vi "QImaging_Main.vi"() -> ()   [LabVIEW 2014]
uses:
  QImaging_Basic/Controls/Parameter.ctl
  Release/QImaging.dll
  QImaging_Basic/Controls/Readout Speed.ctl
panel:
  out "dy":dbl
  in  "Readout Speed":T1
  out "Message":string
  in  "Stop Live Preview":bool
  in  "Abort Multi Grab":bool
  in  "Multi Grab":bool
  out "Saturating?":bool
  out "Average":dbl
  out "Std Dev":dbl
  in  "Overwrite?":bool
  in  "Snap current Data":bool
  in  "Save Data":bool
  in  "Racine chemin de sauvegarde":path=path "C:/Users/loa/Documents/DONNEES MANIP GAZ/Hiver 2015"
  out "Warning":bool
  out "Message":string
  in  "Indice":u32
  in  "Nom":string="tir"
  in  "Mode de Sauvegarde":u16(ring)=1 items=["Manuel", "Automatique"]
  out "Max Val":u16
  out "Captured Image":u16[][](graph)
  out "CCD Height":u32=1 min=1 max=4 step=1
  out "CCD Width":u32=1 min=1 max=4 step=1
  out "Camera Handle":u32
  in  "Abort Frame":bool
  out "sizeOfBuf":u32
  out "errcode":i32
  out "pBuf address":u32
  out "pFrame address":u32
  out "Waiting for Trigger":bool
  in  "Grab Image":bool
  in  "Queue Frame":bool
  in  "Trig":bool
  out "ROI Height":u32=1 min=1 max=4 step=1
  out "ROI Width":u32=1 min=1 max=4 step=1
  in  "Binning":u32=1 min=1 max=4 step=1
  out "ParamVal":u32[](array[numeric])
  out "Open Cam Error":i32
  out "LibCam Error":u32
  out "LibOpen error":i32
  in  "Exposure Time (µs)":u32=100
  out "Camera Id":u32
  out "error out":errorcluster
  in  "error in (no error)":errorcluster
  in  "Stop":bool
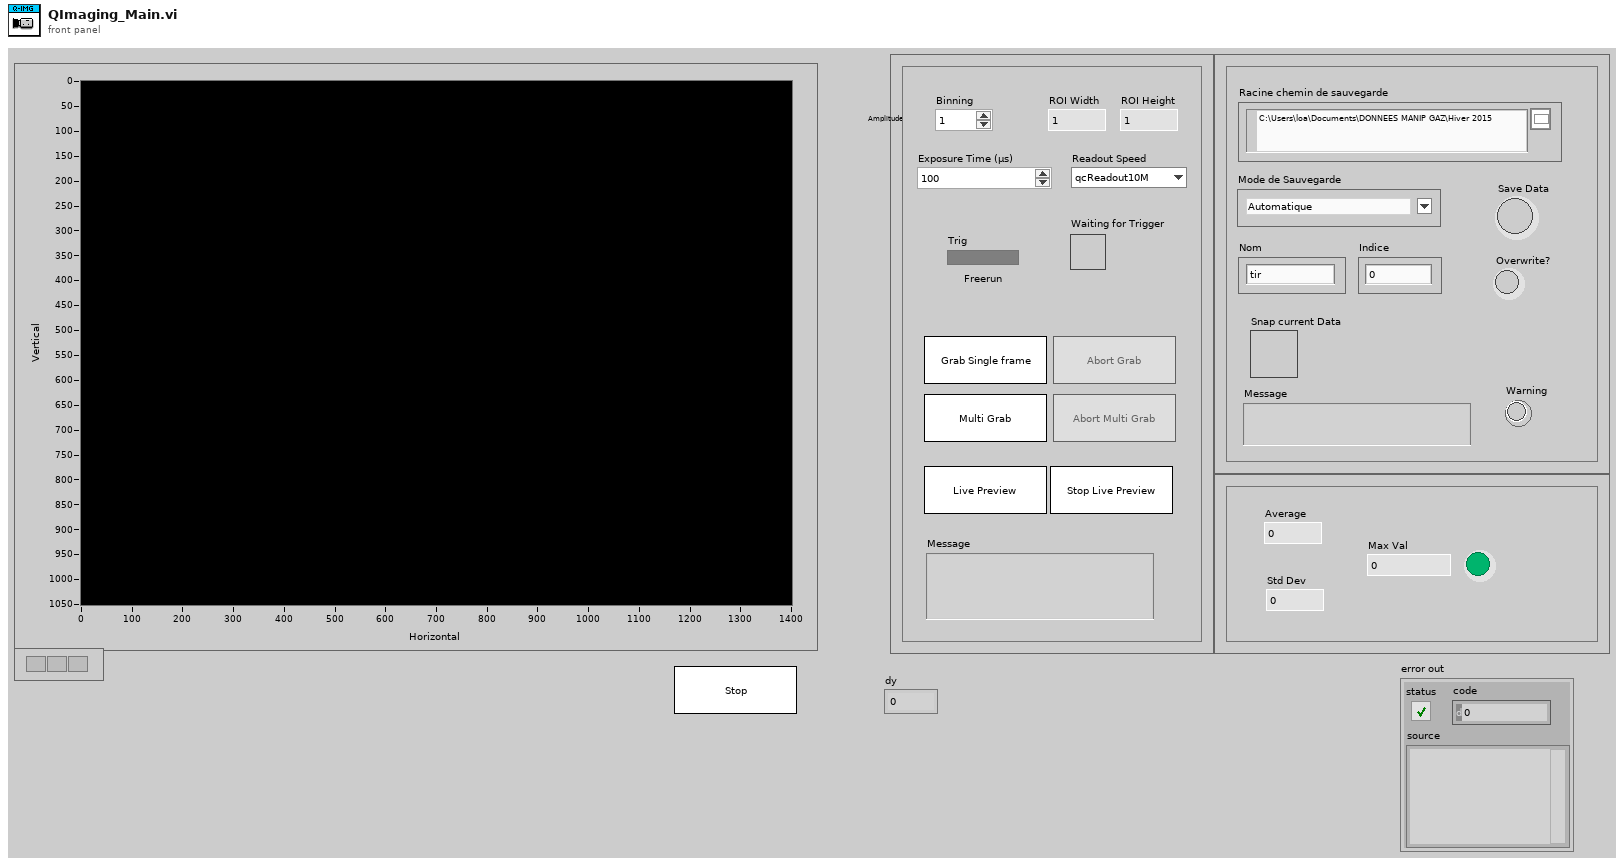
[diagram p1: front panel]
types:
  T1 = typedef "Readout Speed.ctl" = enum16{"qcReadout10M", "qcReadout20M", "qcReadout30M"}
  T2 = enum8{"Enabled", "Disabled", "Disabled and Grayed Out"}
  T3 = typedef "Parameter.ctl" = enum32{"Gain ", "Offset", "Exposure", "Binning", "HzBinning", "VtBinning", "Readout speed", "Trigger Type", "Color Wheel", "Cooler Active", "Exposure red", "Exposure blue", "Image format", "ROI X", "ROI Y", "ROI Width", "ROI Height", "Reserved1", "Shutter State", "Reserved2", "SyncB", "Reserved3", "IntensifierGain (deprecated)", "Trig Delay", "Camera Mode", "Normalized Gain", "Normalized Intensifier Gain", "Do post processing ", "Post Proc Gain Red", "Post Proc Gain Green", "Post Proc Gain Blue", "Post Proc Bayer Algo", "Post Proc Image Format", "Fan Speed", "Blackout Mode", "High Sensitivity Mode", "Readout Port", "EM Gain", "Open Delay Shutter", "Close Delay Shutter", "CCD Clearing Mode", "Over Sample", "Reserved5", "Reserved6", "Reserved7"}
  T4 = typedef "Image Type" = u32
  T5 = typedef "IMAQ Image.ctl" = refnum<image>
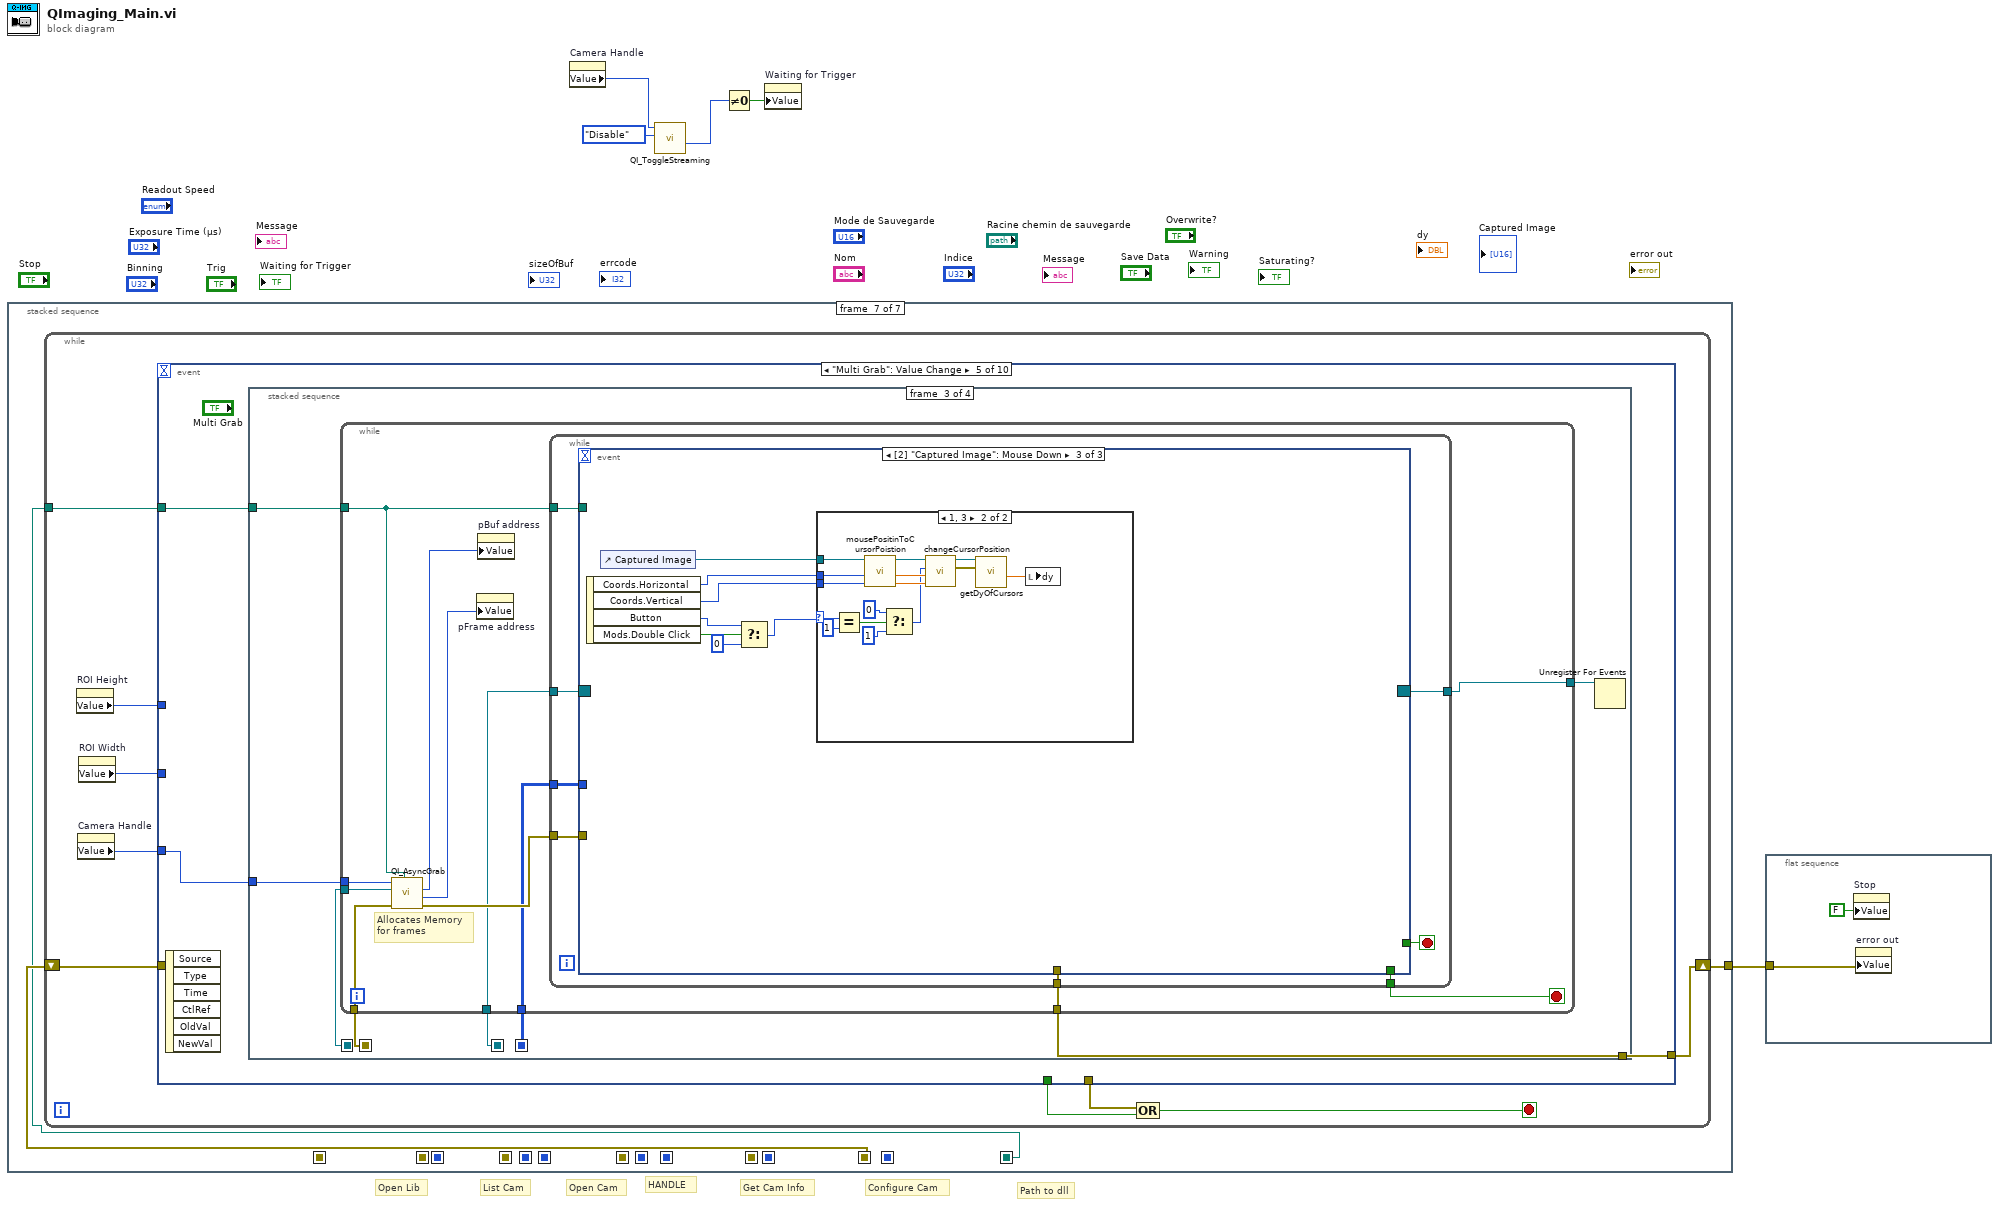
[diagram p0: block diagram]
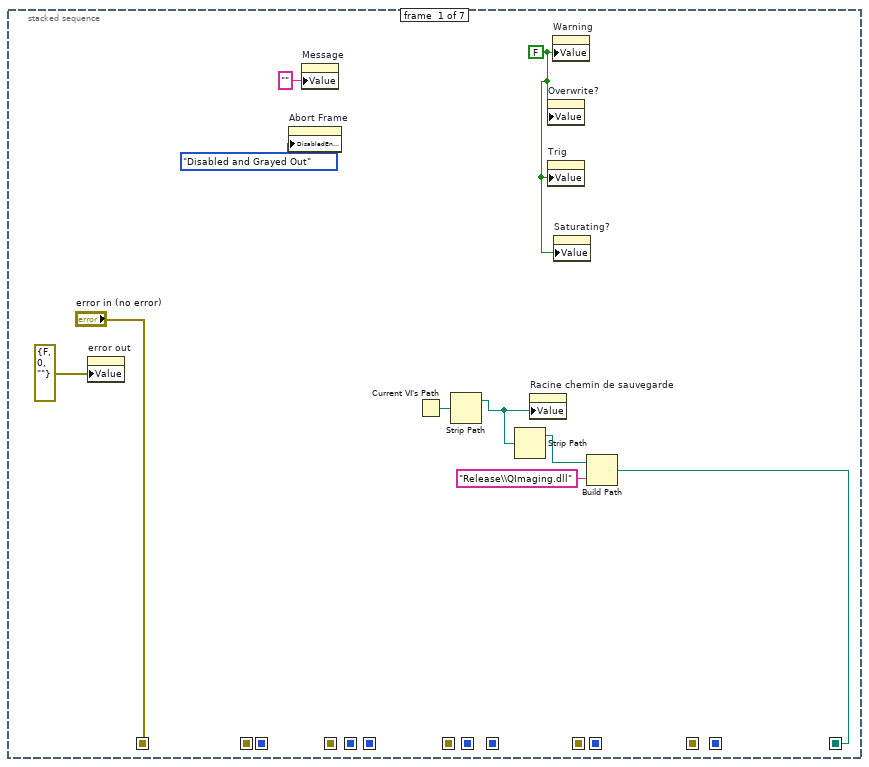
[diagram p2: hidden frame]
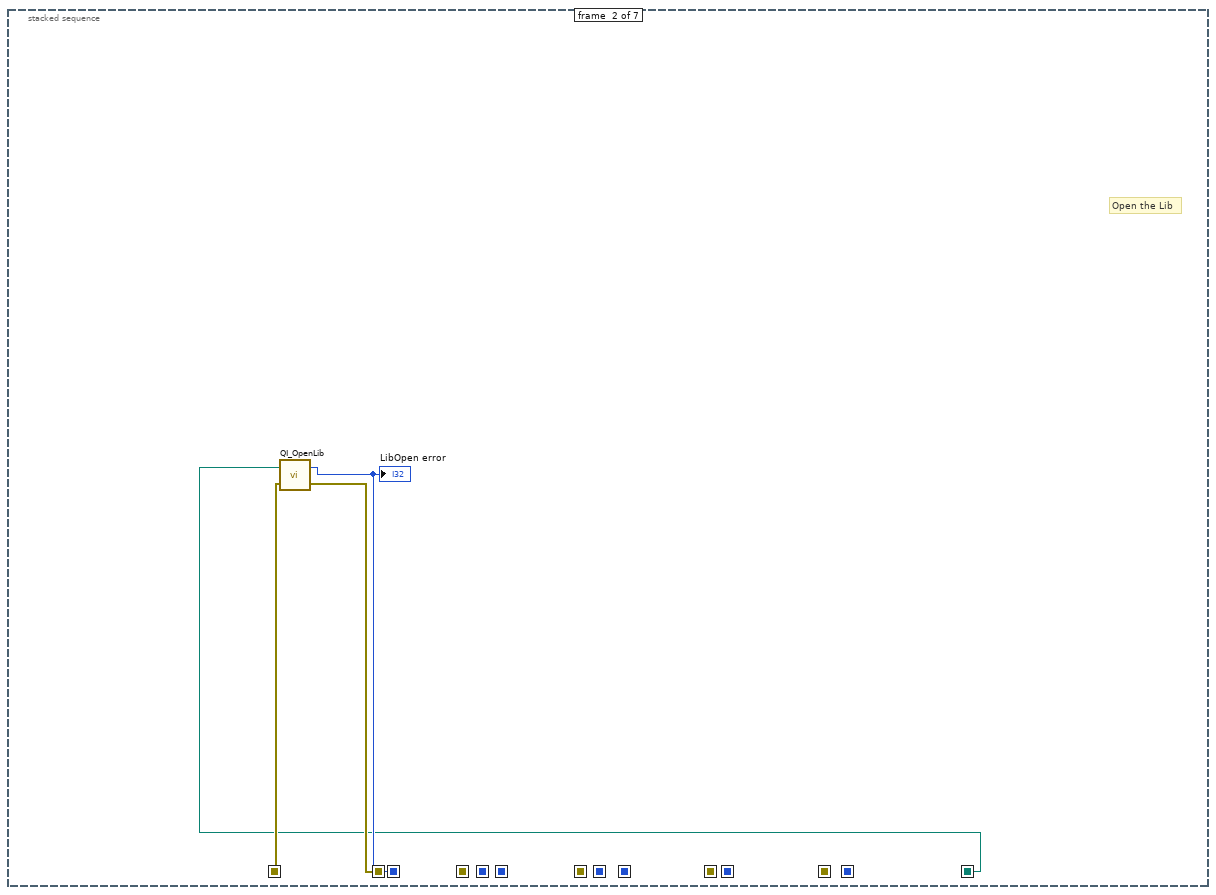
[diagram p3: hidden frame]
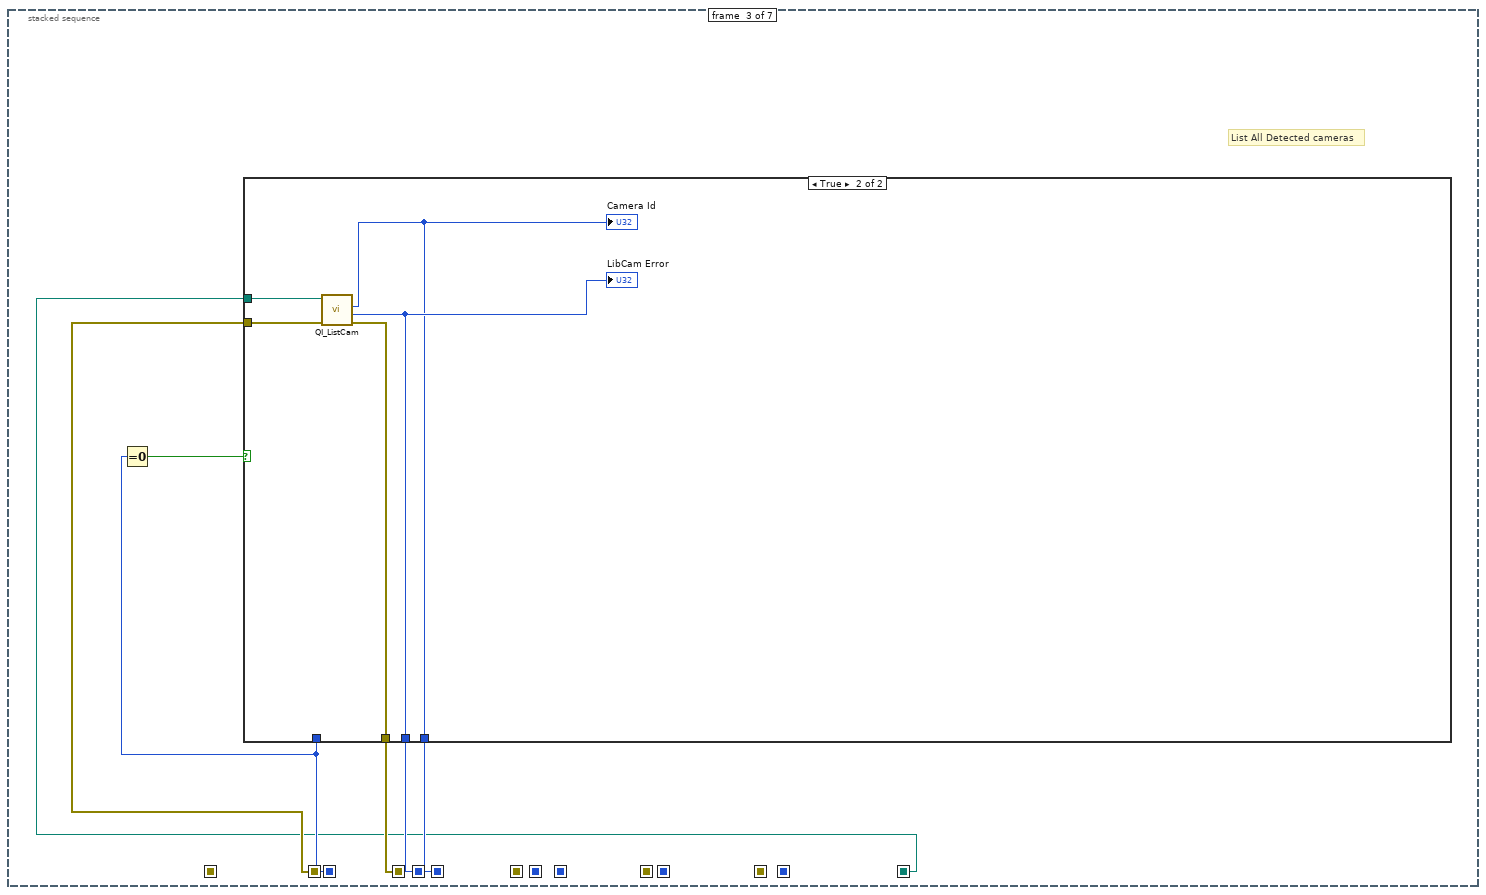
[diagram p4: hidden frame]
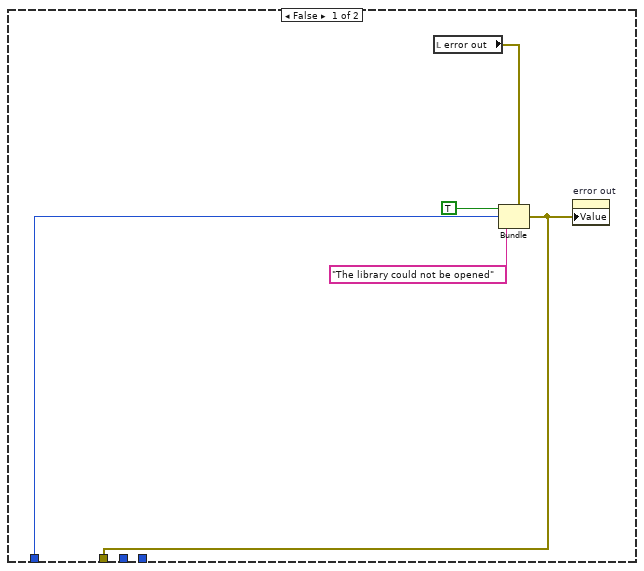
[diagram p5: hidden frame]
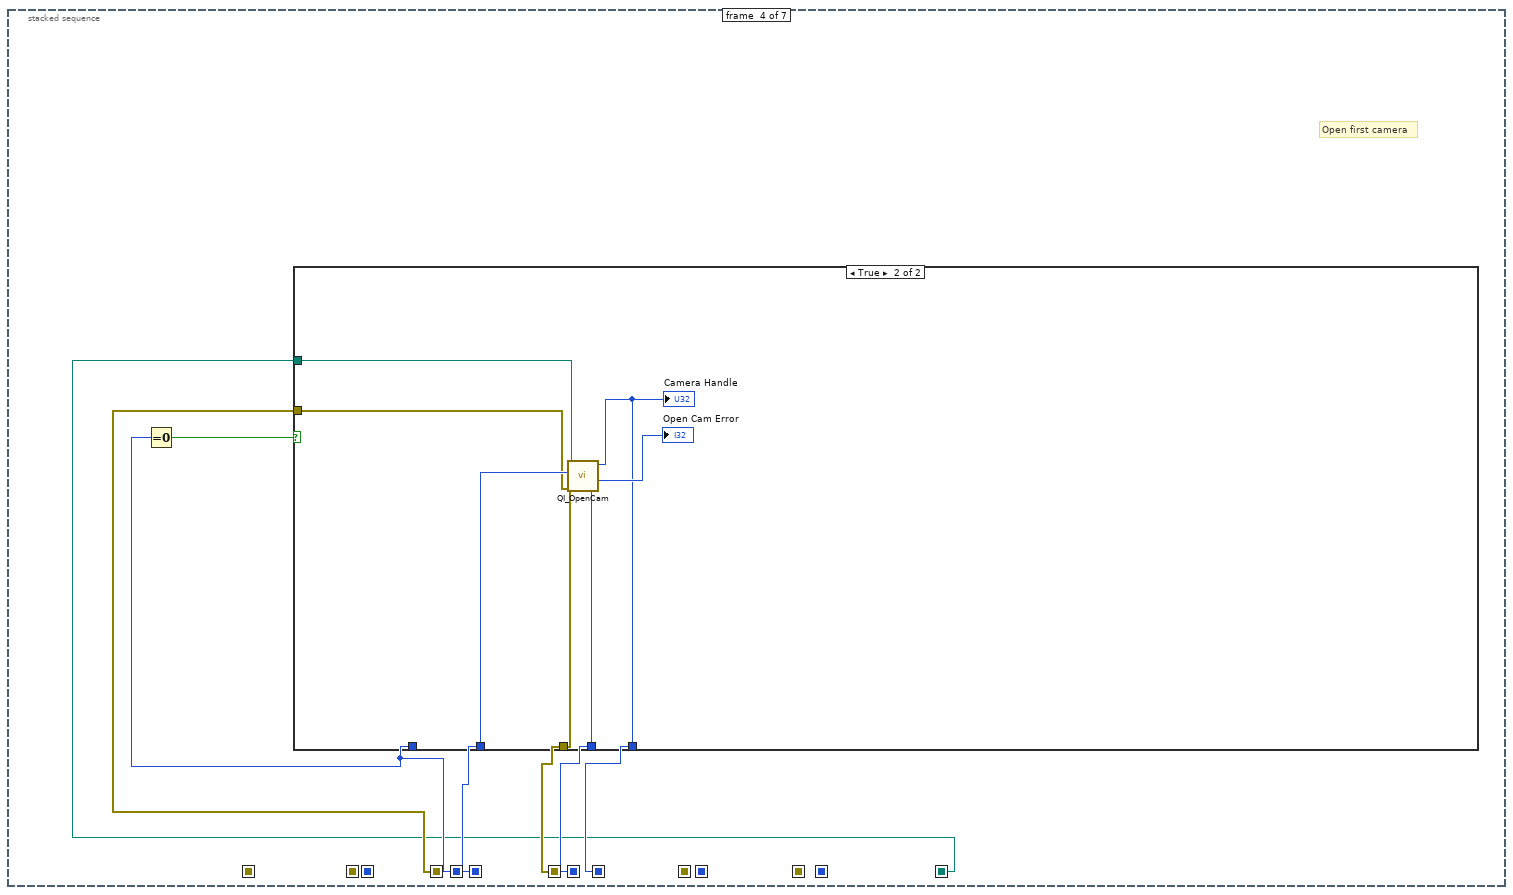
[diagram p6: hidden frame]
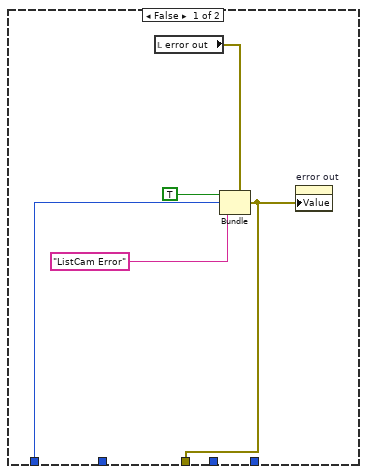
[diagram p7: hidden frame]
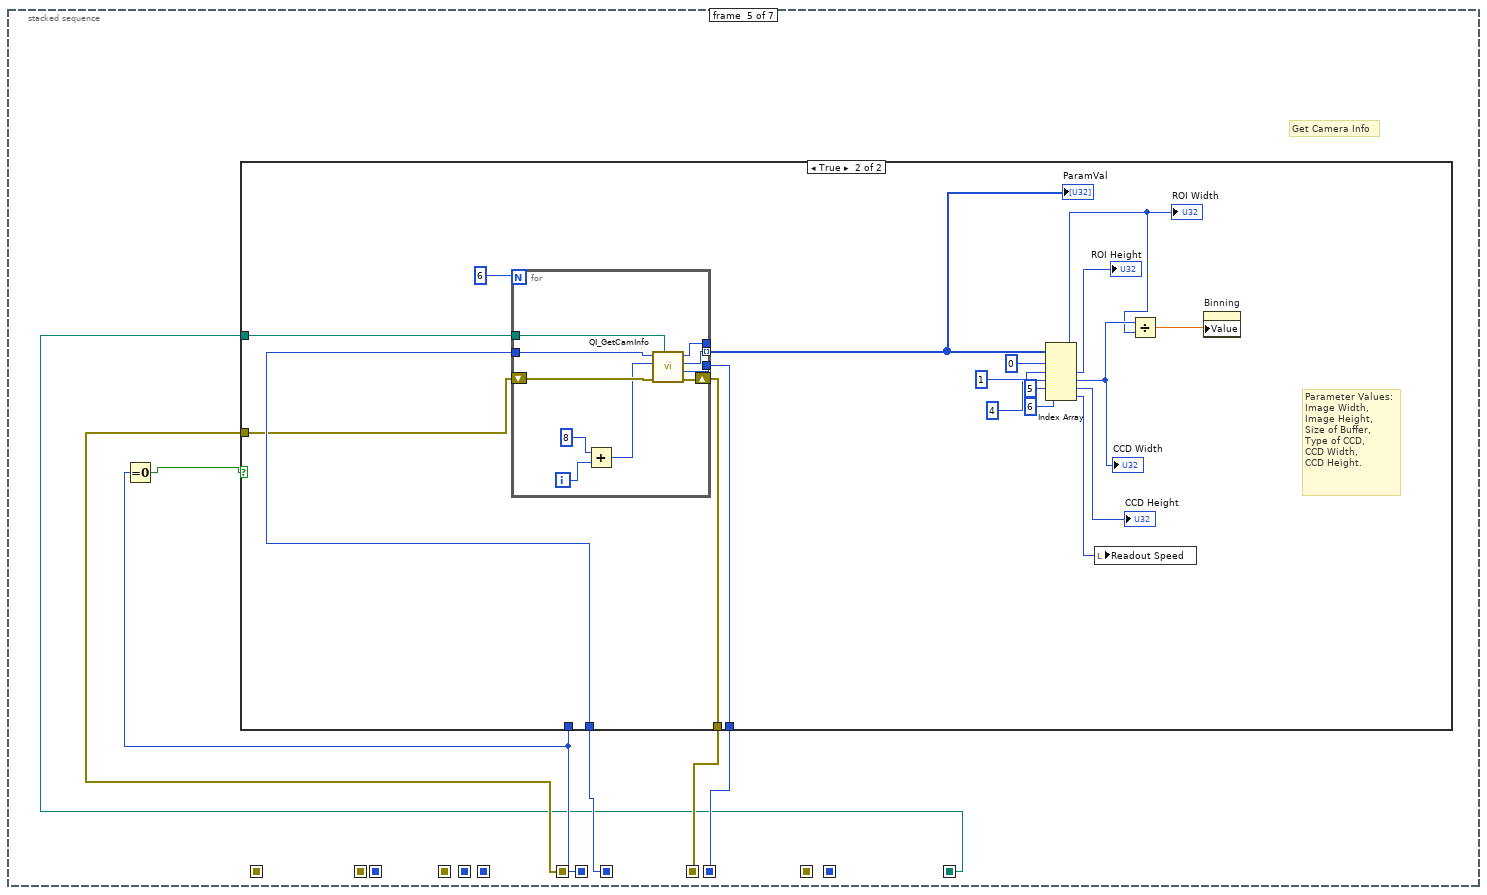
[diagram p8: hidden frame]
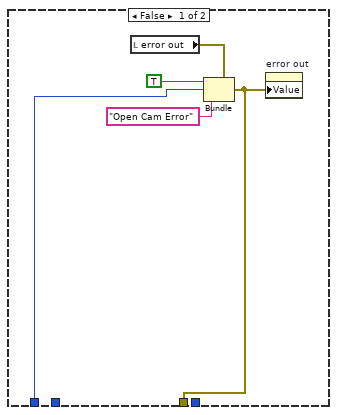
[diagram p9: hidden frame]
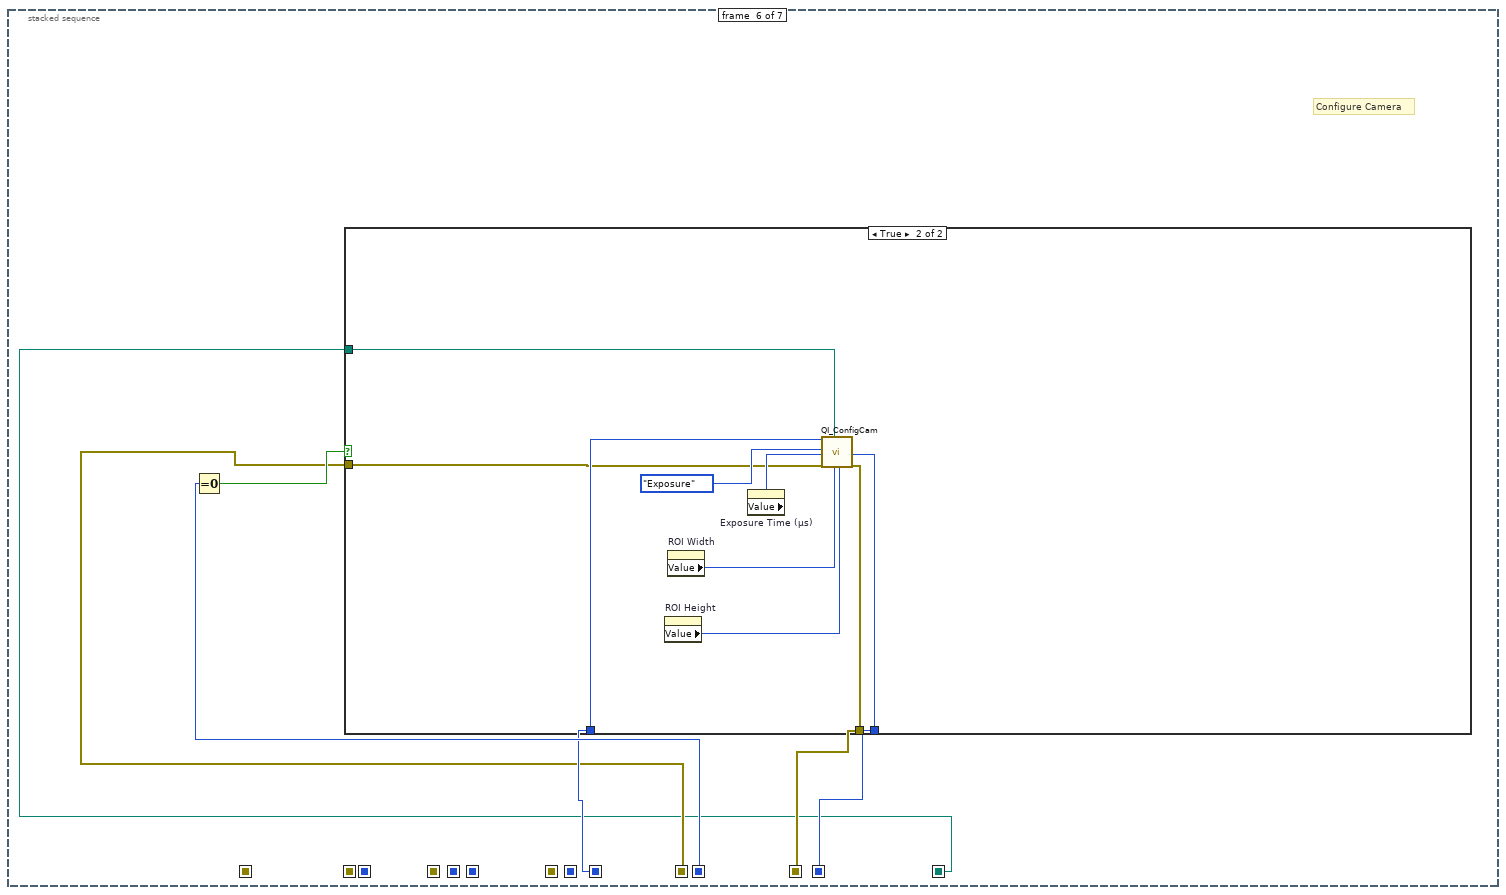
[diagram p10: hidden frame]
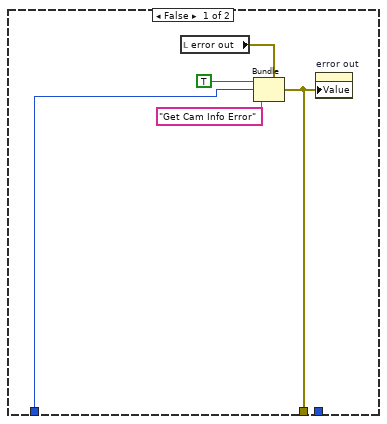
[diagram p11: hidden frame]
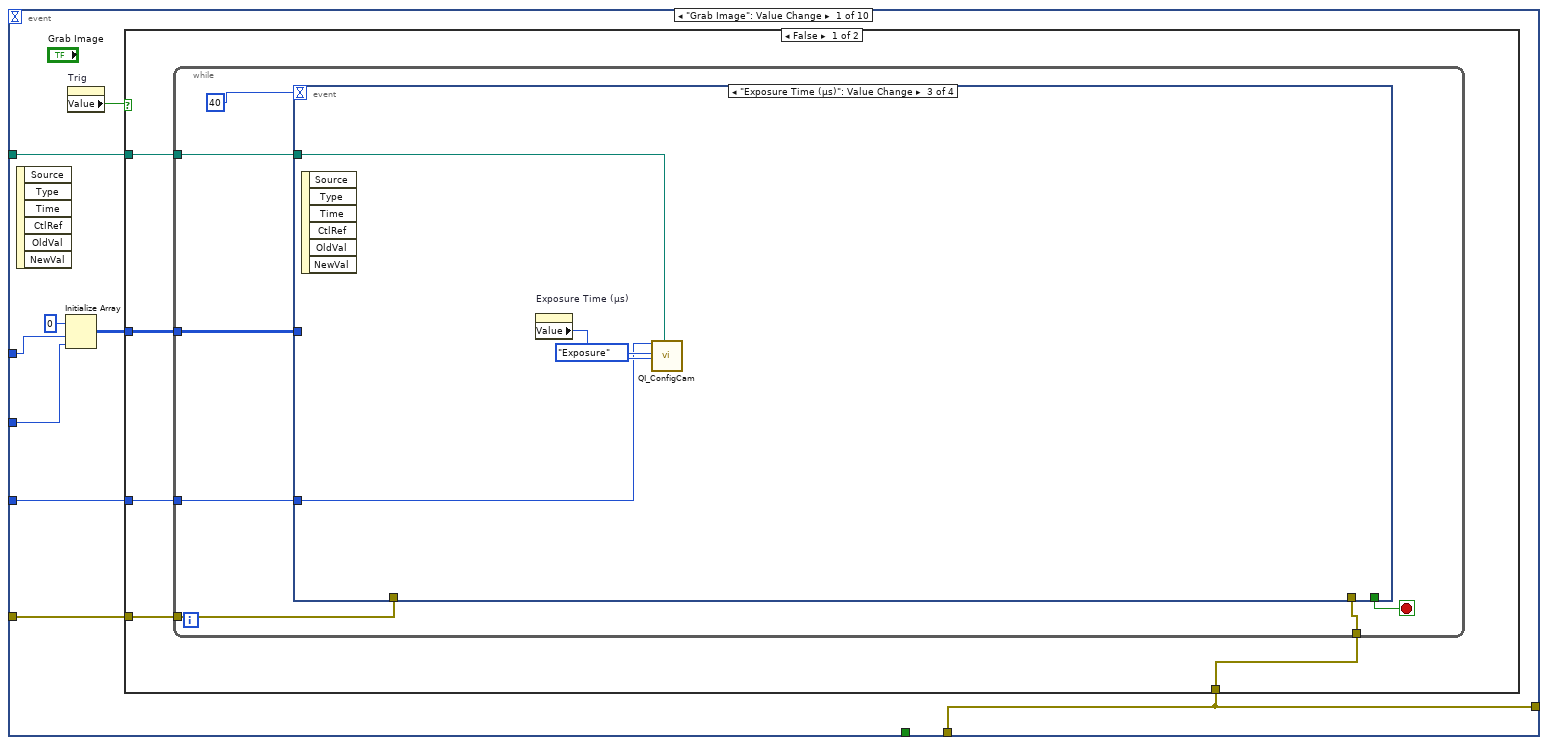
[diagram p12: hidden frame]
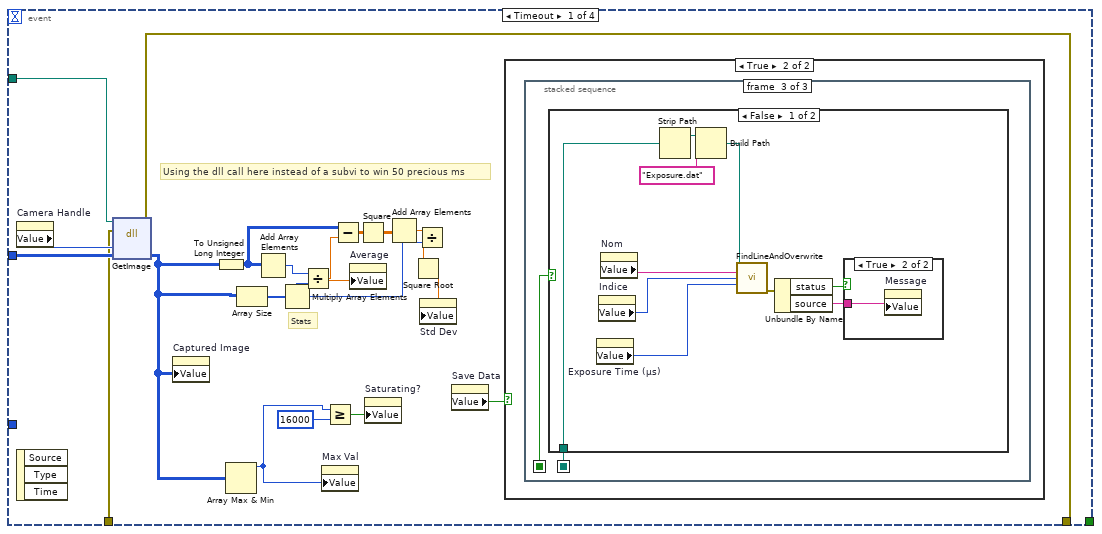
[diagram p13: hidden frame]
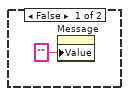
[diagram p14: hidden frame]
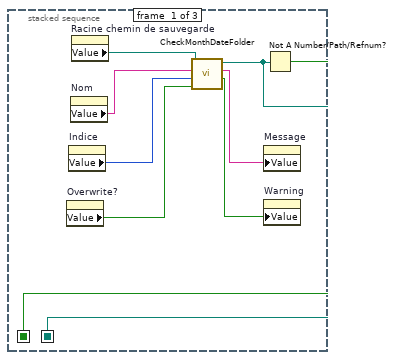
[diagram p15: hidden frame]
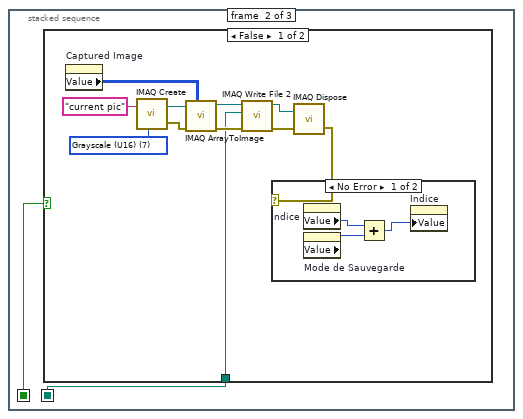
[diagram p16: hidden frame]
diagram:
  # "Path to dll"
  # "HANDLE"
  # "Configure Cam"
  # "Get Cam Info"
  # "Open Cam"
  # "List Cam"
  # "Open Lib"
  n1 = stacked-sequence {
    seq-local: [_ w19 _ _ _ _ _] -> [_ _ w21 _ _ _ _]
    seq-local: [_ w18 _ _ _ _ _] -> [_ _ w23 _ _ _ _]
    seq-local: [_ _ w26 _ _ _ _] -> [_ _ _ w38 _ _ _]
    seq-local: [_ _ w25 _ _ _ _] -> [_ _ _ w40 _ _ _]
    seq-local: [_ _ w24 _ _ _ _] -> [_ _ _ w44 _ _ _]
    seq-local: [_ _ _ w43 _ _ _] -> [_ _ _ _ w57 _ _]
    seq-local: [_ _ _ w42 _ _ _] -> [_ _ _ _ w59 _ _]
    seq-local: [_ _ _ w41 _ _ _] -> [_ _ _ _ w62 w101 _]
    seq-local: [_ _ _ _ w61 _ _] -> [_ _ _ _ _ w97 _]
    seq-local: [_ _ _ _ w60 _ _] -> [_ _ _ _ _ w102 _]
    seq-local: [_ _ _ _ _ w100 _] -> [_ _ _ _ _ _ w119]
    seq-local: [_ _ _ _ _ w99 _] -> [_ _ _ _ _ _ _]
    seq-local: ["error in (no error)" _ _ _ _ _ _] -> [_ w17 _ _ _ _ _]
    seq-local: [w6 _ _ _ _ _ _] -> [_ w16 w20 w37 w56 w96 w117]
    tunnel: [_ _ _ _ _ _ w118] -> w5
    frame #0 {
      w11 = FALSE ("Warning")
      n2 = property on="error out" class="Clust (strict)"("Value"=errorcluster {"status"=FALSE, "code"=0, "source"=""} ("error in (no error)")) -> ()  [unwired: 2 in, 2 out]
      n3 = property on="Abort Frame" class="Bool"("DisabledEnum"=T2."Disabled and Grayed Out" ("Disabled")) -> ()  [unwired: 2 in, 2 out]
      n4 = property on="Message" class="Str"("Value"="" ("Message")) -> ()  [unwired: 2 in, 2 out]
      n5 = Current VI's Path() -> (path=w10:path)
      n6 = Strip Path(path=w10) -> (stripped path=w9:path)  [unwired: 1 out]
      n7 = Strip Path(path=w9) -> (stripped path=w8:path)  [unwired: 1 out]
      n8 = property on="Racine chemin de sauvegarde" class="Path"("Value"=w9) -> ()  [unwired: 2 in, 2 out]
      n9 = property on="Overwrite?" class="Bool (strict)"("Value"=w11) -> ()  [unwired: 2 in, 2 out]
      n10 = property on="Trig" class="Bool (strict)"("Value"=w11) -> ()  [unwired: 2 in, 2 out]
      n11 = property on="Warning" class="Bool (strict)"("Value"=w11) -> ()  [unwired: 2 in, 2 out]
      n12 = property on="Saturating?" class="Bool (strict)"("Value"=w11) -> ()  [unwired: 2 in, 2 out]
      n13 = Build Path(base path=w8, name or relative path="Release\\QImaging.dll") -> (appended path=w6:path)
    }
    frame #1 {
      # "Open the Lib"
      n14 = call "QI_OpenLib.vi"("error in (no error)"=w17, "path to dll"=w16) -> ("error out"=w19:errorcluster, "LibOpen error"=w18:i32)
      "LibOpen error" <- w18
    }
    frame #2 {
      # "List All Detected cameras"
      n15 = Equal To 0?(x=w23) -> (x = 0?=w22:bool)
      n16 = case shown="True" w22 {
        tunnel: w23 -> [w28 _]
        tunnel: [w27 w36] -> w26
        tunnel: [_ w35] -> w25
        tunnel: [_ w34] -> w24
        tunnel: w21 -> [_ w33]
        tunnel: w20 -> [_ w32]
        frame False {
          n17 = local read "error out"() -> (w29:errorcluster)
          n18 = Bundle(cluster=w29, "status"=TRUE, "code"=w28, "source"="The library could not be opened") -> (w27:errorcluster)
          n19 = property on="error out" class="Clust (strict)"("Value"=w27) -> ()  [unwired: 2 in, 2 out]
        }
        frame True {
          n20 = call "QI_ListCam.vi"("error in (no error)"=w33, "path to dll"=w32) -> ("error out"=w36:errorcluster, "LibCam Error"=w35:u32, "cameraId"=w34:u32)  [unwired: 7 in]
          "Camera Id" <- w34
          "LibCam Error" <- w35
        }
      }
    }
    frame #3 {
      # "Open first camera"
      n21 = Equal To 0?(x=w40) -> (x = 0?=w39:bool)
      n22 = case shown="True" w39 {
        tunnel: w44 -> [_ w55]
        tunnel: [w45 w54] -> w43
        tunnel: [_ w53] -> w42
        tunnel: [_ w52] -> w41
        tunnel: w40 -> [w46 _]
        tunnel: w38 -> [_ w51]
        tunnel: w37 -> [_ w50]
        frame False {
          n23 = local read "error out"() -> (w47:errorcluster)
          n24 = Bundle(cluster=w47, "status"=TRUE, "code"=w46, "source"="ListCam Error") -> (w45:errorcluster)
          n25 = property on="error out" class="Clust (strict)"("Value"=w45) -> ()  [unwired: 2 in, 2 out]
        }
        frame True {
          n26 = call "QI_OpenCam.vi"("error in (no error)"=w51, "Camera ID"=w55, "path to dll"=w50) -> ("error out"=w54:errorcluster, "Open Cam Error"=w53:i32, "Camera Handle"=w52:u32)  [unwired: 6 in]
          "Camera Handle" <- w52
          "Open Cam Error" <- w53
        }
      }
    }
    frame #4 {
      # "Get Camera Info"
      n27 = Equal To 0?(x=w59) -> (x = 0?=w58:bool)
      n28 = case shown="True" w58 {
        tunnel: w62 -> [_ w81]
        tunnel: [w63 w80] -> w61
        tunnel: w59 -> [w64 _]
        tunnel: [_ w79] -> w60
        tunnel: w57 -> [_ w78]
        tunnel: w56 -> [_ w73]
        frame False {
          n29 = local read "error out"() -> (w65:errorcluster)
          n30 = Bundle(cluster=w65, "status"=TRUE, "code"=w64, "source"="Open Cam Error") -> (w63:errorcluster)
          n31 = property on="error out" class="Clust (strict)"("Value"=w63) -> ()  [unwired: 2 in, 2 out]
        }
        frame True {
          # "Parameter Values:\nImage Width,\nImage Height,\nSize of Buffer,\nType of CCD,\nCCD Width,\nCCD Height."
          n32 = for {
            N: 6 -> [_]
            shift-right: [w91] -> w80
            shift-left: w78 -> [w95]
            tunnel: [w90] -> _
            tunnel: [w89] -> w83 mode=indexing
            tunnel: [w88] -> w79
            tunnel: w81 -> [w87]
            tunnel: w73 -> [w86]
            i -> [w94]
            n33 = Add(x=u32 8, y=w94) -> (x+y=w92:u32)
            n34 = call "QI_GetCamInfo.vi"("path to dll"=w86, "error in (no error)"=w95, "paramKey"=w92, "Camera Handle"=w87) -> ("error out"=w91:errorcluster, "CamInfo err"=w88:i32, "paramVal"=w89:u32, "Camera Handle"=w90:u32)  [unwired: 4 in]
          }
          "ParamVal" <- w83
          n35 = Index Array(array=w83, index #1=0 ("index"), index #2=1 ("index"), index #3=4 ("index"), index #4=5 ("index"), index #5=6 ("index")) -> (element #1=w71:u32, element #2=→"ROI Height":u32, element #3=w72:u32, element #4=→"CCD Height":u32, element #5=w68:u32)
          "ROI Width" <- w71
          "CCD Width" <- w72
          n36 = local write "Readout Speed"(w68) -> ()
          n37 = Divide(x=w72, y=w71) -> (x/y=w70:dbl)
          n38 = property on="Binning" class="DigNum (strict)"("Value"=w70) -> ()  [unwired: 2 in, 2 out]
        }
      }
    }
    frame #5 {
      # "Configure Camera"
      n39 = Equal To 0?(x=w102) -> (x = 0?=w98:bool)
      n40 = case shown="True" w98 {
        tunnel: w101 -> [w104 w114]
        tunnel: [w103 w111] -> w100
        tunnel: [_ w110] -> w99
        tunnel: w97 -> [_ w109]
        tunnel: w96 -> [_ w108]
        frame False {
          n41 = local read "error out"() -> (w105:errorcluster)
          n42 = Bundle(cluster=w105, "status"=TRUE, "code"=w104, "source"="Get Cam Info Error") -> (w103:errorcluster)
          n43 = property on="error out" class="Clust (strict)"("Value"=w103) -> ()  [unwired: 2 in, 2 out]
        }
        frame True {
          n44 = property on="ROI Height" class="DigNum (strict)"() -> ("Value"=w112:u32)  [unwired: 2 in, 2 out]
          n45 = property on="ROI Width" class="DigNum (strict)"() -> ("Value"=w113:u32)  [unwired: 2 in, 2 out]
          n46 = property on="Exposure Time (µs)" class="DigNum (strict)"() -> ("Value"=w115:u32)  [unwired: 2 in, 2 out]
          n47 = call "QI_ConfigCam.vi"("Camera Handle"=w114, "Parameter"=Parameter."Exposure", "paramVal"=w115, "error in (no error)"=w109, "path to dll"=w108, "CCD Width"=w113, "CCD Height"=w112) -> ("ConfigCam err"=w110:i32, "error out"=w111:errorcluster)  [unwired: 10 in, 1 out]
        }
      }
    }
    frame #6 {
      n48 = while {
        shift-right: [w127] -> w118
        shift-left: w119 -> [w128]
        tunnel: w117 -> [w120]
        stop <- w123 stop-if-true
        n49 = property on="ROI Height" class="DigNum (strict)"() -> ("Value"=w125:u32)  [unwired: 2 in, 2 out]
        n50 = property on="Camera Handle" class="DigNum (strict)"() -> ("Value"=w126:u32)  [unwired: 2 in, 2 out]
        n51 = property on="ROI Width" class="DigNum (strict)"() -> ("Value"=w124:u32)  [unwired: 2 in, 2 out]
        n52 = event shown="[4] \"Multi Grab\": Value Change" {
          selector: _ -> [_ _ _ _ _ _ _ _ _ _]
          dyn-events: _ -> [_ _ _ _ _ _ _ _ _ _]
          timeout: _ -> [_ _ _ _ _ _ _ _ _ _]
          tunnel: w128 -> [w137 _ _ w265 _ _ w540 w559 w576 _]
          tunnel: [w136 w216 _ w263 w378 _ w539 w558 w573 _] -> w127
          tunnel: w126 -> [w135 w218 _ w266 w377 w533 w541 w560 w574 _]
          tunnel: w125 -> [w132 _ _ _ _ _ _ _ _ _]
          tunnel: w124 -> [w131 _ _ _ _ _ _ _ _ _]
          tunnel: [w136 _ _ _ _ w532 w539 w558 w573 _] -> w122
          tunnel: [_ _ _ _ _ TRUE _ _ _ _] -> w121
          tunnel: w120 -> [w129 w219 _ w257 w376 w530 w538 w544 w572 _]
          event "Grab Image": Value Change {
            n53 = event-data() -> ()  [unwired: 1 in, 6 out]
            n54 = Initialize Array(u16 0 ("element"), w132, w131) -> (w130:u16[][])
            n55 = property on="Trig" class="Bool (strict)"() -> ("Value"=w134:bool)  [unwired: 2 in, 2 out]
            n56 = case shown="False" w134 {
              tunnel: w137 -> [w142 w214]
              tunnel: [w139 w214] -> w136
              tunnel: w135 -> [w141 _]
              tunnel: w130 -> [w140 _]
              tunnel: w129 -> [w138 _]
              frame False {
                n57 = while {
                  tunnel: w142 -> [w149]
                  tunnel: w141 -> [w148]
                  tunnel: w140 -> [w145]
                  tunnel: [w144] -> w139
                  tunnel: w138 -> [w143]
                  stop <- w146 stop-if-true
                  n58 = event shown="[2] \"Exposure Time (µs)\": Value Change" {
                    selector: _ -> [_ _ _ _]
                    dyn-events: _ -> [_ _ _ _]
                    timeout: 40 -> [_ _ _ _]
                    tunnel: w149 -> [w153 _ _ _]
                    tunnel: w148 -> [_ _ w210 _]
                    tunnel: [_ TRUE _ TRUE] -> w146
                    tunnel: w145 -> [w158 _ _ _]
                    tunnel: [w151 _ _ _] -> w144
                    tunnel: w143 -> [w152 _ w209 _]
                    event Timeout {
                      # "Using the dll call here instead of a subvi to win 50 precious ms"
                      # "Stats"
                      n59 = property on="Camera Handle" class="DigNum (strict)"() -> ("Value"=w159:u32)  [unwired: 2 in, 2 out]
                      n60 = event-data() -> ()  [unwired: 1 in, 3 out]
                      n61 = dll-call lib="C:/Users/appli/Documents/Aline/octo-labview/QImaging/Release/QImaging.dll" fn="GetImage"(path in=w152, error in=w153, "handle"=w159, "data"=w158) -> (error out=w151:errorcluster, "data"=w154:u16[][])  [unwired: 3 in, 1 out]
                      n62 = property on="Captured Image" class="IntGraph (strict)"("Value"=w154) -> ()  [unwired: 2 in, 2 out]
                      n63 = To Unsigned Long Integer(number=w154) -> (unsigned 32bit integer=w156:u32[][])
                      n64 = Array Max & Min(array=w154) -> (max value=w160:u16)  [unwired: 3 out]
                      n65 = Array Size(array=w154) -> (size(s)=w157:i32[])
                      n66 = Add Array Elements(numeric array=w156) -> (sum=w165:u32)
                      n67 = Multiply Array Elements(1:w157) -> (0:w167:i32)
                      n68 = Divide(x=w165, y=w167) -> (x/y=w162:dbl)
                      n69 = property on="Max Val" class="DigNum (strict)"("Value"=w160) -> ()  [unwired: 2 in, 2 out]
                      n70 = Greater Or Equal?(x=w160, y=u16 16000) -> (x >= y?=w163:bool)
                      n71 = Subtract(x=w156, y=w162) -> (x-y=w169:dbl[][])
                      n72 = property on="Average" class="DigNum (strict)"("Value"=w162) -> ()  [unwired: 2 in, 2 out]
                      n73 = Square(x=w169) -> (x^2=w155:dbl[][])
                      n74 = property on="Saturating?" class="Bool (strict)"("Value"=w163) -> ()  [unwired: 2 in, 2 out]
                      n75 = Add Array Elements(numeric array=w155) -> (sum=w168:dbl)
                      n76 = Divide(x=w168, y=w167) -> (x/y=w166:dbl)
                      n77 = Square Root(x=w166) -> (sqrt(x)=w161:dbl)
                      n78 = property on="Std Dev" class="DigNum (strict)"("Value"=w161) -> ()  [unwired: 2 in, 2 out]
                      n79 = property on="Save Data" class="Bool (strict)"() -> ("Value"=w150:bool)  [unwired: 2 in, 2 out]
                      n80 = case shown="True" w150 {
                        frame False {
                          n81 = property on="Message" class="Str"("Value"="" ("Message Acquisition")) -> ()  [unwired: 2 in, 2 out]
                        }
                        frame True {
                          n82 = stacked-sequence {
                            seq-local: [w172 _ _] -> [_ w180 w196]
                            seq-local: [w171 _ _] -> [_ w179 w195]
                            frame #0 {
                              n83 = property on="Overwrite?" class="Bool (strict)"() -> ("Value"=w173:bool)  [unwired: 2 in, 2 out]
                              n84 = property on="Indice" class="DigNum (strict)"() -> ("Value"=w176:u32)  [unwired: 2 in, 2 out]
                              n85 = property on="Nom" class="Str"() -> ("Value"=w177:string)  [unwired: 2 in, 2 out]
                              n86 = property on="Racine chemin de sauvegarde" class="Path"() -> ("Value"=w178:path)  [unwired: 2 in, 2 out]
                              n87 = call "CheckMonthDateFolder.vi"("Overwrite?"=w173, "Index"=w176, "File Name"=w177, "Folder Path Control"=w178) -> ("Warning"=w174:bool, "Message"=w175:string, "File Path"=w171:path)  [unwired: 5 in]
                              n88 = property on="Message" class="Str"("Value"=w175) -> ()  [unwired: 2 in, 2 out]
                              n89 = property on="Warning" class="Bool (strict)"("Value"=w174) -> ()  [unwired: 2 in, 2 out]
                              n90 = Not A Number/Path/Refnum?(number/path/refnum=w171) -> (NaN/Path/Refnum?=w172:bool)
                            }
                            frame #1 {
                              n91 = case shown="False" w180 {
                                tunnel: w179 -> [w182 _]
                                frame False {
                                w187 = T4 7 items=["Grayscale (U8)", "Grayscale (I16)", "Grayscale (SGL)", "Complex (CSG)", "RGB (U32)", "HSL (U32)", "RGB (U64)", "Grayscale (U16)"] ("Image Type")
                                n92 = property on="Captured Image" class="IntGraph (strict)"() -> ("Value"=w183:u16[][])  [unwired: 2 in, 2 out]
                                n93 = call "IMAQ Create"("Image Name"="current pic", "Image Type"=w187) -> ("New Image"=w190:T5, "error out"=w184:errorcluster)  [unwired: 3 in]
                                n94 = call "IMAQ ArrayToImage"("Image Pixels (U16)"=w183, "error in (no error)"=w184, "Image"=w190) -> ("error out"=w185:errorcluster, "Image Out"=w191:T5)  [unwired: 7 in]
                                n95 = call-poly "IMAQ Write File 2"("error in (no error)"=w185, "File Path"=w182, "Image"=w191) -> ("error out"=w186:errorcluster, "Image Out (duplicate)"=w189:T5)  [unwired: 7 in]
                                n96 = call "IMAQ Dispose"("Image"=w189, "error in (no error)"=w186) -> ("error out"=w181:errorcluster)  [unwired: 4 in]
                                n97 = case shown="No Error" w181 {
                                frame No Error {
                                n98 = property on="Indice" class="DigNum (strict)"() -> ("Value"=w194:u32)  [unwired: 2 in, 2 out]
                                n99 = property on="Mode de Sauvegarde" class="Ring (strict)"() -> ("Value"=w193:u16)  [unwired: 2 in, 2 out]
                                n100 = Add(x=w194, y=w193) -> (x+y=w192:u32)
                                n101 = property on="Indice" class="DigNum (strict)"("Value"=w192) -> ()  [unwired: 2 in, 2 out]
                                }
                                frame Error {
                                }
                                }
                                }
                                frame True {
                                }
                              }
                            }
                            frame #2 {
                              n102 = case shown="False" w196 {
                                tunnel: w195 -> [w204 _]
                                frame False {
                                n103 = property on="Exposure Time (µs)" class="DigNum (strict)"() -> ("Value"=w201:u32)  [unwired: 2 in, 2 out]
                                n104 = property on="Indice" class="DigNum (strict)"() -> ("Value"=w202:u32)  [unwired: 2 in, 2 out]
                                n105 = property on="Nom" class="Str"() -> ("Value"=w203:string)  [unwired: 2 in, 2 out]
                                n106 = Strip Path(path=w204) -> (stripped path=w205:path)  [unwired: 1 out]
                                n107 = Build Path(base path=w205, name or relative path="Exposure.dat" ("Image Name")) -> (appended path=w197:path)
                                n108 = call "FindLineAndOverwrite.vi"("File Path"=w197, "Name"=w203, "Index"=w202, "Exposure"=w201) -> ("error out"=w200:errorcluster)  [unwired: 11 in]
                                n109 = Unbundle By Name(w200) -> ("status"=w199:bool, "source"=w198:string)
                                n110 = case shown="True" w199 {
                                tunnel: w198 -> [_ w207]
                                frame False {
                                }
                                frame True {
                                n111 = property on="Message" class="Str"("Value"=w207) -> ()  [unwired: 2 in, 2 out]
                                }
                                }
                                }
                                frame True {
                                }
                              }
                            }
                          }
                        }
                      }
                    }
                    event "Stop Live Preview": Value Change {
                      n112 = event-data() -> ()  [unwired: 1 in, 6 out]
                    }
                    event "Exposure Time (µs)": Value Change {
                      n113 = event-data() -> ()  [unwired: 1 in, 6 out]
                      n114 = property on="Exposure Time (µs)" class="DigNum (strict)"() -> ("Value"=w211:u32)  [unwired: 2 in, 2 out]
                      n115 = call "QI_ConfigCam.vi"("Camera Handle"=w210, "Parameter"=Parameter."Exposure", "paramVal"=w211, "path to dll"=w209) -> ()  [unwired: 13 in, 3 out]
                    }
                    event "Stop": Value Change {
                      n116 = event-data() -> ()  [unwired: 1 in, 6 out]
                    }
                  }
                }
              }
              frame True {
                n117 = property on="Message" class="Str"("Value"="This function is not available when the camera trig is hardware. Use Multi Grab or Grab Single Frame instead. " ("Message Acquisition")) -> ()  [unwired: 2 in, 2 out]
              }
            }
          }
          event Value Change {
            n118 = event-data() -> ()  [unwired: 1 in, 6 out]
            n119 = local read "Readout Speed"() -> (w217:T1)
            n120 = call "QI_ConfigCam.vi"("Camera Handle"=w218, "Parameter"=Parameter."Readout speed", "Readout Speed"=w217, "path to dll"=w219) -> ("error out"=w216:errorcluster)  [unwired: 13 in, 2 out]
          }
          event "Snap current Data": Value Change {
            n121 = event-data() -> ()  [unwired: 1 in, 6 out]
            n122 = property on="Overwrite?" class="Bool (strict)"() -> ("Value"=w223:bool)  [unwired: 2 in, 2 out]
            n123 = property on="Indice" class="DigNum (strict)"() -> ("Value"=w226:u32)  [unwired: 2 in, 2 out]
            n124 = property on="Nom" class="Str"() -> ("Value"=w227:string)  [unwired: 2 in, 2 out]
            n125 = property on="Racine chemin de sauvegarde" class="Path"() -> ("Value"=w228:path)  [unwired: 2 in, 2 out]
            n126 = call "CheckMonthDateFolder.vi"("Overwrite?"=w223, "Index"=w226, "File Name"=w227, "Folder Path Control"=w228) -> ("Warning"=w224:bool, "Message"=w225:string, "File Path"=w221:path)  [unwired: 5 in]
            n127 = property on="Message" class="Str"("Value"=w225) -> ()  [unwired: 2 in, 2 out]
            n128 = property on="Warning" class="Bool (strict)"("Value"=w224) -> ()  [unwired: 2 in, 2 out]
            n129 = Not A Number/Path/Refnum?(number/path/refnum=w221) -> (NaN/Path/Refnum?=w222:bool)
            n130 = case shown="False" w222 {
              tunnel: w221 -> [w229 _]
              frame False {
                n131 = stacked-sequence {
                  seq-local: [w232 _ _] -> [_ _ w252]
                  tunnel: w229 -> [w231 w244 _]
                  frame #0 {
                    w236 = T4 7 items=["Grayscale (U8)", "Grayscale (I16)", "Grayscale (SGL)", "Complex (CSG)", "RGB (U32)", "HSL (U32)", "RGB (U64)", "Grayscale (U16)"] ("Image Type")
                    n132 = property on="Captured Image" class="IntGraph (strict)"() -> ("Value"=w230:u16[][])  [unwired: 2 in, 2 out]
                    n133 = call "IMAQ Create"("Image Name"="current pic", "Image Type"=w236) -> ("New Image"=w239:T5, "error out"=w233:errorcluster)  [unwired: 3 in]
                    n134 = call "IMAQ ArrayToImage"("Image Pixels (U16)"=w230, "error in (no error)"=w233, "Image"=w239) -> ("error out"=w234:errorcluster, "Image Out"=w240:T5)  [unwired: 7 in]
                    n135 = call-poly "IMAQ Write File 2"("error in (no error)"=w234, "File Path"=w231, "Image"=w240) -> ("error out"=w235:errorcluster, "Image Out (duplicate)"=w238:T5)  [unwired: 7 in]
                    n136 = call "IMAQ Dispose"("Image"=w238, "error in (no error)"=w235) -> ("error out"=w232:errorcluster)  [unwired: 4 in]
                  }
                  frame #1 {
                    # "Write exposure file"
                    n137 = property on="Exposure Time (µs)" class="DigNum (strict)"() -> ("Value"=w246:u32)  [unwired: 2 in, 2 out]
                    n138 = property on="Indice" class="DigNum (strict)"() -> ("Value"=w247:u32)  [unwired: 2 in, 2 out]
                    n139 = property on="Nom" class="Str"() -> ("Value"=w248:string)  [unwired: 2 in, 2 out]
                    n140 = Strip Path(path=w244) -> (stripped path=w249:path)  [unwired: 1 out]
                    n141 = Build Path(base path=w249, name or relative path="Exposure.dat" ("Image Name")) -> (appended path=w245:path)
                    n142 = call "FindLineAndOverwrite.vi"("File Path"=w245, "Name"=w248, "Index"=w247, "Exposure"=w246) -> ("error out"=w241:errorcluster)  [unwired: 11 in]
                    n143 = Unbundle By Name(w241) -> ("status"=w243:bool, "source"=w242:string)
                    n144 = case shown="True" w243 {
                      tunnel: w242 -> [_ w251]
                      frame False {
                      }
                      frame True {
                        n145 = property on="Message" class="Str"("Value"=w251) -> ()  [unwired: 2 in, 2 out]
                      }
                    }
                  }
                  frame #2 {
                    n146 = case shown="No Error" w252 {
                      frame No Error {
                        n147 = property on="Mode de Sauvegarde" class="Ring (strict)"() -> ("Value"=w254:u16)  [unwired: 2 in, 2 out]
                        n148 = property on="Indice" class="DigNum (strict)"() -> ("Value"=w255:u32)  [unwired: 2 in, 2 out]
                        n149 = Add(x=w255, y=w254) -> (x+y=w253:u32)
                        n150 = property on="Indice" class="DigNum (strict)"("Value"=w253) -> ()  [unwired: 2 in, 2 out]
                      }
                      frame Error {
                      }
                    }
                  }
                }
              }
              frame True {
              }
            }
          }
          event "Queue Frame": Value Change {
            n151 = event-data() -> ()  [unwired: 1 in, 6 out]
            n152 = call "QI_ToggleStreaming.vi"("path to dll"=w257, "error in (no error)"=w265, "Enable?"=enum16{"Disable", "Enable"}."Enable", "Camera Handle"=w266) -> ("error out"=w268:errorcluster, "enable"=w261:u32, "Camera Handle"=w267:u32)  [unwired: 4 in, 1 out]
            n153 = flat-sequence {
              tunnel: w257 -> [w277]
              tunnel: [w277] -> w256
              frame #0 {
                n154 = property on="Queue Frame" class="Bool"("DisabledEnum"=T2."Disabled and Grayed Out" ("Disabled")) -> ()  [unwired: 2 in, 2 out]
                n155 = property on="Abort Frame" class="Bool"("DisabledEnum"=T2."Enabled" ("Disabled")) -> ()  [unwired: 2 in, 2 out]
              }
            }
            n156 = Not Equal To 0?(x=w261) -> (x != 0?=w262:bool)
            n157 = Create User Event(user event datatype="" ("stringMessage")) -> (user event=w271:refnum<user-event>)  [unwired: 1 in, 1 out]
            n158 = property on="Waiting for Trigger" class="Bool (strict)"("Value"=w262) -> ()  [unwired: 2 in, 2 out]
            n159 = register-events(w271) -> (reference out=w274:refnum<event-registration>)  [unwired: 2 in, 1 out]
            n160 = call "QI_AsyncGrab.vi"("path to dll"=w257, "error in (no error)"=w268, "UserEventRef"=w271, "Camera Handle"=w267) -> ("error out"=w269:errorcluster, "Frame Address"=→"pFrame address":u32, "Buffer Address"=→"pBuf address":u32)  [unwired: 4 in, 1 out]
            n161 = property on="ROI Width" class="DigNum (strict)"() -> ("Value"=w259:u32)  [unwired: 2 in, 2 out]
            n162 = property on="ROI Height" class="DigNum (strict)"() -> ("Value"=w260:u32)  [unwired: 2 in, 2 out]
            n163 = Initialize Array(u16 0 ("element"), w260, w259) -> (w272:u16[][])
            n164 = while {
              tunnel: w274 -> [w285]
              tunnel: w272 -> [w282]
              tunnel: w269 -> [w281]
              tunnel: [w280] -> w263
              tunnel: w256 -> [w279]
              stop <- w283 stop-if-true
              n165 = event shown="[1] \"Abort Frame\": Value Change" {
                selector: w285 -> [_ _]
                dyn-events: [_ _] -> w284
                timeout: _ -> [_ _]
                tunnel: [TRUE TRUE] -> w283
                tunnel: w282 -> [w288 _]
                tunnel: w281 -> [w287 w373]
                tunnel: [w286 w368] -> w280
                tunnel: w279 -> [_ w364]
                event User Event {
                  n166 = event-data() -> ()  [unwired: 1 in, 1 out]
                  n167 = stacked-sequence {
                    seq-local: [_ w291 _ _ _ _] -> [_ _ _ _ w304 w349]
                    tunnel: w288 -> [_ w294 _ _ _ _]
                    tunnel: w287 -> [_ _ _ w301 _ _]
                    tunnel: [_ _ _ w300 _ _] -> w286
                    frame #0 {
                      # "Wait until image is available from driver"
                      n168 = Wait (ms)(milliseconds to wait=u32 200) -> ()  [unwired: 1 out]
                    }
                    frame #1 {
                      # "Get data to interface"
                      n169 = property on="ROI Width" class="DigNum (strict)"() -> ("Value"=w292:u32)  [unwired: 2 in, 2 out]
                      n170 = property on="ROI Height" class="DigNum (strict)"() -> ("Value"=w293:u32)  [unwired: 2 in, 2 out]
                      n171 = property on="pBuf address" class="DigNum (strict)"() -> ("Value"=w295:u32)  [unwired: 2 in, 2 out]
                      n172 = dll-call lib="Z:/Programmes en Developpement/QImaging/Release/QImaging.dll" fn="GetFrame"("width"=w292, "height"=w293, "pBuf"=w295, "data"=w294) -> ("data"=w291:u16[][])  [unwired: 7 in, 2 out]
                      n173 = property on="Captured Image" class="IntGraph (strict)"("Value"=w291) -> ()  [unwired: 2 in, 2 out]
                    }
                    frame #2 {
                      # "ALWAYS free memory\nafter calling Async Grab\n(calls malloc)"
                      n174 = property on="pBuf address" class="DigNum (strict)"() -> ("Value"=w296:u32)  [unwired: 2 in, 2 out]
                      n175 = property on="pFrame address" class="DigNum (strict)"() -> ("Value"=w297:u32)  [unwired: 2 in, 2 out]
                      n176 = dll-call lib="Z:/Programmes en Developpement/QImaging/Release/QImaging.dll" fn="RemFrame"("pFrame"=w297, "pBuf"=w296) -> ()  [unwired: 6 in, 2 out]
                    }
                    frame #3 {
                      # "Disable Streaming"
                      n177 = property on="Camera Handle" class="DigNum (strict)"() -> ("Value"=w302:u32)  [unwired: 2 in, 2 out]
                      n178 = call "QI_ToggleStreaming.vi"("error in (no error)"=w301, "Enable?"=enum16{"Disable", "Enable"}."Disable", "Camera Handle"=w302) -> ("error out"=w300:errorcluster, "enable"=w298:u32)  [unwired: 5 in, 2 out]
                      n179 = Not Equal To 0?(x=w298) -> (x != 0?=w299:bool)
                      n180 = property on="Waiting for Trigger" class="Bool (strict)"("Value"=w299) -> ()  [unwired: 2 in, 2 out]
                    }
                    frame #4 {
                      # "Save data"
                      n181 = property on="Save Data" class="Bool (strict)"() -> ("Value"=w305:bool)  [unwired: 2 in, 2 out]
                      n182 = case shown="True" w305 {
                        tunnel: w304 -> [_ w311]
                        frame False {
                        }
                        frame True {
                          n183 = property on="Indice" class="DigNum (strict)"() -> ("Value"=w314:u32)  [unwired: 2 in, 2 out]
                          n184 = property on="Overwrite?" class="Bool (strict)"() -> ("Value"=w315:bool)  [unwired: 2 in, 2 out]
                          n185 = property on="Nom" class="Str"() -> ("Value"=w313:string)  [unwired: 2 in, 2 out]
                          n186 = property on="Racine chemin de sauvegarde" class="Path"() -> ("Value"=w312:path)  [unwired: 2 in, 2 out]
                          n187 = call "CheckMonthDateFolder.vi"("Overwrite?"=w315, "Index"=w314, "File Name"=w313, "Folder Path Control"=w312) -> ("Warning"=w317:bool, "Message"=w316:string, "File Path"=w306:path)  [unwired: 5 in]
                          n188 = property on="Message" class="Str"("Value"=w316) -> ()  [unwired: 2 in, 2 out]
                          n189 = property on="Warning" class="Bool (strict)"("Value"=w317) -> ()  [unwired: 2 in, 2 out]
                          n190 = Strip Path(path=w306) -> (stripped path=w307:path)  [unwired: 1 out]
                          n191 = Build Path(base path=w307, name or relative path="Exposure.dat" ("Image Name")) -> (appended path=w308:path)
                          n192 = Not A Number/Path/Refnum?(number/path/refnum=w306) -> (NaN/Path/Refnum?=w310:bool)
                          n193 = case shown="False" w310 {
                            tunnel: w311 -> [w320 _]
                            tunnel: w306 -> [w321 _]
                            tunnel: w308 -> [w319 _]
                            tunnel: w306 -> [w318 _]
                            frame False {
                              n194 = stacked-sequence {
                                seq-local: [w330 _] -> [_ w341]
                                tunnel: w321 -> [w329 _]
                                tunnel: w320 -> [w331 _]
                                tunnel: w319 -> [w328 _]
                                tunnel: w318 -> [_ _]
                                frame #0 {
                                w335 = T4 7 items=["Grayscale (U8)", "Grayscale (I16)", "Grayscale (SGL)", "Complex (CSG)", "RGB (U32)", "HSL (U32)", "RGB (U64)", "Grayscale (U16)"] ("Image Type")
                                n195 = property on="Exposure Time (µs)" class="DigNum (strict)"() -> ("Value"=w325:u32)  [unwired: 2 in, 2 out]
                                n196 = property on="Indice" class="DigNum (strict)"() -> ("Value"=w326:u32)  [unwired: 2 in, 2 out]
                                n197 = property on="Nom" class="Str"() -> ("Value"=w327:string)  [unwired: 2 in, 2 out]
                                n198 = call "FindLineAndOverwrite.vi"("File Path"=w328, "Name"=w327, "Index"=w326, "Exposure"=w325) -> ("error out"=w324:errorcluster)  [unwired: 11 in]
                                n199 = Unbundle By Name(w324) -> ("status"=w323:bool, "source"=w322:string)
                                n200 = call "IMAQ Create"("Image Name"="", "Image Type"=w335) -> ("New Image"=w338:T5, "error out"=w332:errorcluster)  [unwired: 3 in]
                                n201 = case shown="True" w323 {
                                tunnel: w322 -> [_ w340]
                                frame False {
                                }
                                frame True {
                                n202 = property on="Message" class="Str"("Value"=w340) -> ()  [unwired: 2 in, 2 out]
                                }
                                }
                                n203 = call "IMAQ ArrayToImage"("Image Pixels (U16)"=w331, "error in (no error)"=w332, "Image"=w338) -> ("error out"=w333:errorcluster, "Image Out"=w339:T5)  [unwired: 7 in]
                                n204 = call-poly "IMAQ Write File 2"("error in (no error)"=w333, "File Path"=w329, "Image"=w339) -> ("error out"=w334:errorcluster, "Image Out (duplicate)"=w337:T5)  [unwired: 7 in]
                                n205 = call "IMAQ Dispose"("Image"=w337, "error in (no error)"=w334) -> ("error out"=w330:errorcluster)  [unwired: 4 in]
                                }
                                frame #1 {
                                n206 = case shown="No Error" w341 {
                                frame No Error {
                                # "incrémente si mode \nautomatique et écriture \nok"
                                n207 = property on="Mode de Sauvegarde" class="Ring (strict)"() -> ("Value"=w343:u16)  [unwired: 2 in, 2 out]
                                n208 = property on="Indice" class="DigNum (strict)"() -> ("Value"=w344:u32)  [unwired: 2 in, 2 out]
                                n209 = Add(x=w344, y=w343) -> (x+y=w342:u32)
                                n210 = property on="Indice" class="DigNum (strict)"("Value"=w342) -> ()  [unwired: 2 in, 2 out]
                                }
                                frame Error {
                                }
                                }
                                }
                              }
                            }
                            frame True {
                            }
                          }
                        }
                      }
                    }
                    frame #5 {
                      # "Stats"
                      n211 = To Unsigned Long Integer(number=w349) -> (unsigned 32bit integer=w351:u32[][])
                      n212 = Array Size(array=w349) -> (size(s)=w352:i32[])
                      n213 = Add Array Elements(numeric array=w351) -> (sum=w353:u32)
                      n214 = Multiply Array Elements(1:w352) -> (0:w356:i32)
                      n215 = Divide(x=w353, y=w356) -> (x/y=w359:dbl)
                      "Average" <- w359
                      n216 = Subtract(x=w351, y=w359) -> (x-y=w358:dbl[][])
                      n217 = Square(x=w358) -> (x^2=w350:dbl[][])
                      n218 = Add Array Elements(numeric array=w350) -> (sum=w357:dbl)
                      n219 = Divide(x=w357, y=w356) -> (x/y=w354:dbl)
                      n220 = Square Root(x=w354) -> (sqrt(x)=→"Std Dev":dbl)
                      n221 = Array Max & Min(array=w349) -> (max value=w348:u16)  [unwired: 3 out]
                      "Max Val" <- w348
                      n222 = Greater Or Equal?(x=w348, y=u16 16000) -> (x >= y?=w346:bool)
                      n223 = property on="Saturating?" class="Bool (strict)"("Value"=w346) -> ()  [unwired: 2 in, 2 out]
                      n224 = property on="Queue Frame" class="Bool"("DisabledEnum"=T2."Enabled" ("Disabled")) -> ()  [unwired: 2 in, 2 out]
                      n225 = property on="Abort Frame" class="Bool"("DisabledEnum"=T2."Disabled and Grayed Out" ("Disabled")) -> ()  [unwired: 2 in, 2 out]
                    }
                  }
                }
                event "Abort Frame": Value Change {
                  n226 = event-data() -> ()  [unwired: 1 in, 6 out]
                  n227 = property on="Camera Handle" class="DigNum (strict)"() -> ("Value"=w374:u32)  [unwired: 2 in, 2 out]
                  n228 = call "QI_AbortFrame.vi"("path to dll"=w364, "error in (no error)"=w373, "Camera Handle"=w374) -> ("error out"=w363:errorcluster, "Camera Handle"=w369:u32)  [unwired: 7 in]
                  n229 = property on="pBuf address" class="DigNum (strict)"() -> ("Value"=w365:u32)  [unwired: 2 in, 2 out]
                  n230 = property on="pFrame address" class="DigNum (strict)"() -> ("Value"=w366:u32)  [unwired: 2 in, 2 out]
                  n231 = dll-call lib="C:/Users/loa/Documents/Programmes LV/Cameras/QImaging/Release/QImaging.dll" fn="RemFrame"(path in=w364, error in=w363, "pFrame"=w366, "pBuf"=w365) -> (error out=w362:errorcluster)  [unwired: 4 in, 1 out]
                  n232 = call "QI_ToggleStreaming.vi"("path to dll"=w364, "error in (no error)"=w362, "Enable?"=enum16{"Disable", "Enable"}."Disable", "Camera Handle"=w369) -> ("error out"=w368:errorcluster, "enable"=w370:u32)  [unwired: 4 in, 2 out]
                  n233 = property on="Abort Frame" class="Bool"("DisabledEnum"=T2."Disabled and Grayed Out" ("Disabled")) -> ()  [unwired: 2 in, 2 out]
                  n234 = property on="Queue Frame" class="Bool"("DisabledEnum"=T2."Enabled" ("Disabled")) -> ()  [unwired: 2 in, 2 out]
                  n235 = Not Equal To 0?(x=w370) -> (x != 0?=w371:bool)
                  n236 = property on="Waiting for Trigger" class="Bool (strict)"("Value"=w371) -> ()  [unwired: 2 in, 2 out]
                }
              }
              n237 = Unregister For Events(event registration refnum=w284) -> ()  [unwired: 1 in, 1 out]
            }
          }
          event "Multi Grab": Value Change {
            n238 = event-data() -> ()  [unwired: 1 in, 6 out]
            n239 = stacked-sequence {
              seq-local: [_ w388 _ _] -> [_ _ w397 _]
              seq-local: [_ w387 _ _] -> [_ _ w396 _]
              seq-local: [_ w386 _ _] -> [_ _ w399 _]
              seq-local: [w380 _ _ _] -> [_ _ w395 _]
              tunnel: [_ _ w400 _] -> w378
              tunnel: w377 -> [_ _ w398 _]
              tunnel: w376 -> [_ _ w393 _]
              frame #0 {
                # "Enable Streaming and grey-out button"
                n240 = property on="Multi Grab" class="Bool"("DisabledEnum"=T2."Disabled and Grayed Out" ("Disabled")) -> ()  [unwired: 2 in, 2 out]
                n241 = property on="Camera Handle" class="DigNum (strict)"() -> ("Value"=w381:u32)  [unwired: 2 in, 2 out]
                n242 = call "QI_ToggleStreaming.vi"("Enable?"=enum16{"Disable", "Enable"}."Enable", "Camera Handle"=w381) -> ("error out"=w380:errorcluster, "enable"=w384:u32)  [unwired: 6 in, 2 out]
                n243 = Not Equal To 0?(x=w384) -> (x != 0?=w383:bool)
                n244 = property on="Waiting for Trigger" class="Bool (strict)"("Value"=w383) -> ()  [unwired: 2 in, 2 out]
              }
              frame #1 {
                # "Register for events (callback) and allocate memory"
                n245 = Create User Event(user event datatype="" ("stringMessage")) -> (user event=w386:refnum<user-event>)  [unwired: 1 in, 1 out]
                n246 = register-events(w386) -> (reference out=w387:refnum<event-registration>)  [unwired: 2 in, 1 out]
                n247 = property on="ROI Width" class="DigNum (strict)"() -> ("Value"=w389:u32)  [unwired: 2 in, 2 out]
                n248 = property on="ROI Height" class="DigNum (strict)"() -> ("Value"=w390:u32)  [unwired: 2 in, 2 out]
                n249 = property on="Abort Multi Grab" class="Bool"("DisabledEnum"=T2."Enabled" ("Disabled")) -> ()  [unwired: 2 in, 2 out]
                n250 = Initialize Array(u16 0 ("element"), w390, w389) -> (w388:u16[][])
              }
              frame #2 {
                n251 = while {
                  tunnel: [w411] -> w400
                  tunnel: w399 -> [w408]
                  tunnel: w398 -> [w407]
                  tunnel: w397 -> [w406]
                  tunnel: w396 -> [w405]
                  tunnel: w395 -> [w404]
                  tunnel: [w403] -> w394
                  tunnel: w393 -> [w401]
                  stop <- w402 stop-if-true
                  # "Allocates Memory\nfor frames"
                  n252 = call "QI_AsyncGrab.vi"("path to dll"=w401, "error in (no error)"=w404, "UserEventRef"=w408, "Camera Handle"=w407) -> ("error out"=w412:errorcluster, "Frame Address"=w409:u32, "Buffer Address"=w410:u32)  [unwired: 4 in, 1 out]
                  n253 = property on="pFrame address" class="DigNum (strict)"("Value"=w409) -> ()  [unwired: 2 in, 2 out]
                  n254 = property on="pBuf address" class="DigNum (strict)"("Value"=w410) -> ()  [unwired: 2 in, 2 out]
                  n255 = while {
                    tunnel: w406 -> [w420]
                    tunnel: w412 -> [w419]
                    tunnel: [w418] -> w411
                    tunnel: w405 -> [w417]
                    tunnel: [w416] -> w403
                    tunnel: [w414] -> w402
                    tunnel: w401 -> [w413]
                    stop <- w415 stop-if-true
                    n256 = event shown="[2] \"Captured Image\": Mouse Down" {
                      selector: w417 -> [_ _ _]
                      dyn-events: [_ _ _] -> w416
                      timeout: _ -> [_ _ _]
                      tunnel: [TRUE w499 _] -> w415
                      tunnel: w420 -> [w424 _ _]
                      tunnel: w419 -> [w423 w496 _]
                      tunnel: [_ w500 _] -> w418
                      tunnel: [FALSE w499 _] -> w414
                      tunnel: w413 -> [w421 w493 _]
                      event User Event {
                        n257 = event-data() -> ()  [unwired: 1 in, 1 out]
                        n258 = stacked-sequence {
                          seq-local: [_ w428 _ _ _] -> [_ _ _ w436 w484]
                          tunnel: w424 -> [_ w432 _ _ _]
                          tunnel: w423 -> [_ _ _ _ _]
                          tunnel: w421 -> [_ w427 w433 _ _]
                          frame #0 {
                            # "Wait until image is available from driver"
                            n259 = Wait (ms)(milliseconds to wait=u32 200) -> ()  [unwired: 1 out]
                          }
                          frame #1 {
                            # "Get data to interface"
                            n260 = property on="pBuf address" class="DigNum (strict)"() -> ("Value"=w429:u32)  [unwired: 2 in, 2 out]
                            n261 = property on="ROI Width" class="DigNum (strict)"() -> ("Value"=w430:u32)  [unwired: 2 in, 2 out]
                            n262 = property on="ROI Height" class="DigNum (strict)"() -> ("Value"=w431:u32)  [unwired: 2 in, 2 out]
                            n263 = dll-call lib="C:/Users/appli/Documents/Aline/octo-labview/QImaging/Release/QImaging.dll" fn="GetFrame"(path in=w427, "width"=w430, "height"=w431, "pBuf"=w429, "data"=w432) -> ("data"=w428:u16[][])  [unwired: 6 in, 2 out]
                            n264 = property on="Captured Image" class="IntGraph (strict)"("Value"=w428) -> ()  [unwired: 2 in, 2 out]
                          }
                          frame #2 {
                            # "ALWAYS free memory\nafter calling Async Grab\n(calls malloc)"
                            n265 = property on="pBuf address" class="DigNum (strict)"() -> ("Value"=w434:u32)  [unwired: 2 in, 2 out]
                            n266 = property on="pFrame address" class="DigNum (strict)"() -> ("Value"=w435:u32)  [unwired: 2 in, 2 out]
                            n267 = dll-call lib="C:/Users/appli/Documents/Aline/octo-labview/QImaging/Release/QImaging.dll" fn="RemFrame"(path in=w433, "pFrame"=w435, "pBuf"=w434) -> ()  [unwired: 5 in, 2 out]
                          }
                          frame #3 {
                            # "Save data"
                            n268 = property on="Save Data" class="Bool (strict)"() -> ("Value"=w437:bool)  [unwired: 2 in, 2 out]
                            n269 = case shown="True" w437 {
                              tunnel: w436 -> [_ w441]
                              frame False {
                              }
                              frame True {
                                n270 = property on="Indice" class="DigNum (strict)"() -> ("Value"=w443:u32)  [unwired: 2 in, 2 out]
                                n271 = property on="Overwrite?" class="Bool (strict)"() -> ("Value"=w444:bool)  [unwired: 2 in, 2 out]
                                n272 = property on="Nom" class="Str"() -> ("Value"=w442:string)  [unwired: 2 in, 2 out]
                                n273 = property on="Racine chemin de sauvegarde" class="Path"() -> ("Value"=w438:path)  [unwired: 2 in, 2 out]
                                n274 = call "CheckMonthDateFolder.vi"("Overwrite?"=w444, "Index"=w443, "File Name"=w442, "Folder Path Control"=w438) -> ("Warning"=w446:bool, "Message"=w445:string, "File Path"=w439:path)  [unwired: 5 in]
                                n275 = property on="Message" class="Str"("Value"=w445) -> ()  [unwired: 2 in, 2 out]
                                n276 = property on="Warning" class="Bool (strict)"("Value"=w446) -> ()  [unwired: 2 in, 2 out]
                                n277 = Not A Number/Path/Refnum?(number/path/refnum=w439) -> (NaN/Path/Refnum?=w440:bool)
                                n278 = case shown="False" w440 {
                                tunnel: w441 -> [w448 _]
                                tunnel: w439 -> [w449 _]
                                tunnel: w438 -> [w447 _]
                                frame False {
                                n279 = stacked-sequence {
                                seq-local: [w450 _ _] -> [_ w461 w465]
                                tunnel: w449 -> [w451 _ _]
                                tunnel: w448 -> [w452 _ _]
                                tunnel: w447 -> [_ _ w470]
                                frame #0 {
                                w456 = T4 7 items=["Grayscale (U8)", "Grayscale (I16)", "Grayscale (SGL)", "Complex (CSG)", "RGB (U32)", "HSL (U32)", "RGB (U64)", "Grayscale (U16)"] ("Image Type")
                                n280 = call "IMAQ Create"("Image Name"="", "Image Type"=w456) -> ("New Image"=w459:T5, "error out"=w453:errorcluster)  [unwired: 3 in]
                                n281 = call "IMAQ ArrayToImage"("Image Pixels (U16)"=w452, "error in (no error)"=w453, "Image"=w459) -> ("error out"=w454:errorcluster, "Image Out"=w460:T5)  [unwired: 7 in]
                                n282 = call-poly "IMAQ Write File 2"("error in (no error)"=w454, "File Path"=w451, "Image"=w460) -> ("error out"=w455:errorcluster, "Image Out (duplicate)"=w458:T5)  [unwired: 7 in]
                                n283 = call "IMAQ Dispose"("Image"=w458, "error in (no error)"=w455) -> ("error out"=w450:errorcluster)  [unwired: 4 in]
                                }
                                frame #1 {
                                n284 = case shown="No Error" w461 {
                                frame No Error {
                                # "incrémente si mode \nautomatique et écriture \nok"
                                n285 = property on="Mode de Sauvegarde" class="Ring (strict)"() -> ("Value"=w463:u16)  [unwired: 2 in, 2 out]
                                n286 = property on="Indice" class="DigNum (strict)"() -> ("Value"=w464:u32)  [unwired: 2 in, 2 out]
                                n287 = Add(x=w464, y=w463) -> (x+y=w462:u32)
                                n288 = property on="Indice" class="DigNum (strict)"("Value"=w462) -> ()  [unwired: 2 in, 2 out]
                                }
                                frame Error {
                                }
                                }
                                }
                                frame #2 {
                                # "Ecrit temps d'expo \ndans fichier de \ndonnées"
                                n289 = property on="Exposure Time (µs)" class="DigNum (strict)"() -> ("Value"=w466:u32)  [unwired: 2 in, 2 out]
                                n290 = property on="Nom" class="Str"() -> ("Value"=w471:string)  [unwired: 2 in, 2 out]
                                n291 = property on="Indice" class="DigNum (strict)"() -> ("Value"=w467:u32)  [unwired: 2 in, 2 out]
                                n292 = Build Path(base path=w470, name or relative path="Exposure.dat") -> (appended path=w468:path)
                                n293 = case shown="No Error" w465 {
                                tunnel: w471 -> [w478 _]
                                tunnel: w468 -> [w477 _]
                                tunnel: w467 -> [w476 _]
                                tunnel: w466 -> [w475 _]
                                frame No Error {
                                n294 = call "FindLineAndOverwrite.vi"("File Path"=w477, "Name"=w478, "Index"=w476, "Exposure"=w475) -> ("error out"=w474:errorcluster)  [unwired: 11 in]
                                n295 = Unbundle By Name(w474) -> ("code"=w473:i32, "source"=w472:string)  [unwired: 1 out]
                                n296 = call <vilib>:"General Error Handler.vi"("[error code] (0)"=w473, "[error source] (\" \")"=w472) -> ()  [unwired: 9 in, 5 out]
                                }
                                frame Error {
                                }
                                }
                                }
                                }
                                }
                                frame True {
                                }
                                }
                              }
                            }
                          }
                          frame #4 {
                            # "Stats"
                            n297 = To Unsigned Long Integer(number=w484) -> (unsigned 32bit integer=w486:u32[][])
                            n298 = Array Size(array=w484) -> (size(s)=w487:i32[])
                            n299 = Add Array Elements(numeric array=w486) -> (sum=w488:u32)
                            n300 = Multiply Array Elements(1:w487) -> (0:w490:i32)
                            n301 = Divide(x=w488, y=w490) -> (x/y=w480:dbl)
                            n302 = Subtract(x=w486, y=w480) -> (x-y=w492:dbl[][])
                            n303 = property on="Average" class="DigNum (strict)"("Value"=w480) -> ()  [unwired: 2 in, 2 out]
                            n304 = Square(x=w492) -> (x^2=w485:dbl[][])
                            n305 = Add Array Elements(numeric array=w485) -> (sum=w491:dbl)
                            n306 = Divide(x=w491, y=w490) -> (x/y=w489:dbl)
                            n307 = Square Root(x=w489) -> (sqrt(x)=w481:dbl)
                            n308 = property on="Std Dev" class="DigNum (strict)"("Value"=w481) -> ()  [unwired: 2 in, 2 out]
                            n309 = Array Max & Min(array=w484) -> (max value=w479:u16)  [unwired: 3 out]
                            n310 = property on="Max Val" class="DigNum (strict)"("Value"=w479) -> ()  [unwired: 2 in, 2 out]
                            n311 = Greater Or Equal?(x=w479, y=u16 16000) -> (x >= y?=w482:bool)
                            n312 = property on="Saturating?" class="Bool (strict)"("Value"=w482) -> ()  [unwired: 2 in, 2 out]
                          }
                        }
                      }
                      event "Abort Multi Grab": Value Change {
                        w499 = TRUE
                        n313 = event-data() -> ()  [unwired: 1 in, 6 out]
                        n314 = property on="Camera Handle" class="DigNum (strict)"() -> ("Value"=w505:u32)  [unwired: 2 in, 2 out]
                        n315 = call "QI_AbortFrame.vi"("path to dll"=w493, "error in (no error)"=w496, "Camera Handle"=w505) -> ("error out"=w495:errorcluster, "Camera Handle"=w501:u32)  [unwired: 7 in]
                        n316 = property on="pFrame address" class="DigNum (strict)"() -> ("Value"=w498:u32)  [unwired: 2 in, 2 out]
                        n317 = property on="pBuf address" class="DigNum (strict)"() -> ("Value"=w497:u32)  [unwired: 2 in, 2 out]
                        n318 = dll-call lib="C:/Users/appli/Documents/Aline/octo-labview/QImaging/Release/QImaging.dll" fn="RemFrame"(path in=w493, error in=w495, "pFrame"=w498, "pBuf"=w497) -> (error out=w494:errorcluster)  [unwired: 4 in, 1 out]
                        n319 = call "QI_ToggleStreaming.vi"("path to dll"=w493, "error in (no error)"=w494, "Enable?"=enum16{"Disable", "Enable"}."Disable", "Camera Handle"=w501) -> ("error out"=w500:errorcluster, "enable"=w502:u32)  [unwired: 4 in, 2 out]
                        n320 = Not Equal To 0?(x=w502) -> (x != 0?=w503:bool)
                        n321 = property on="Waiting for Trigger" class="Bool (strict)"("Value"=w503) -> ()  [unwired: 2 in, 2 out]
                      }
                      event "Captured Image": Mouse Down {
                        n322 = event-data() -> ("Coords.Horizontal"=w507:i32, "Coords.Vertical"=w506:i32, "Button"=w511:u16, "Mods.Double Click"=w512:bool)  [unwired: 1 in]
                        n323 = control-ref of="Captured Image"() -> (w508:refnum<vi>)
                        n324 = Select(t=w511, s=w512, f=u16 0) -> (s? t:f=w509:u16)
                        n325 = case shown="1, 3" w509 {
                          selector: w509 -> [_ w524]
                          tunnel: w508 -> [_ w527]
                          tunnel: w507 -> [_ w526]
                          tunnel: w506 -> [_ w525]
                          frame Default {
                          }
                          frame 1, 3 {
                            n326 = Equal?(x=w524, y=u16 1) -> (x = y?=w523:bool)
                            n327 = call "mousePositinToCursorPoistion.vi"("Mouse Y position"=w525, "Mouse X position"=w526, "reference"=w527) -> ("Cursor Y position"=w519:dbl, "Cursor X position"=w518:dbl, "reference out"=w517:refnum<vi>)  [unwired: 1 in, 1 out]
                            n328 = Select(t=u16 0, s=w523, f=u16 1) -> (s? t:f=w516:u16)
                            n329 = call "changeCursorPosition.vi"("Cursor Y position"=w519, "Cursor X position"=w518, "Cursos id"=w516, "reference"=w517) -> ("error out"=w515:errorcluster, "reference out"=w514:refnum<vi>)  [unwired: 2 in]
                            n330 = call "getDyOfCursors.vi"("error in (no error)"=w515, "reference"=w514) -> ("dy"=w513:dbl)  [unwired: 7 in, 2 out]
                            n331 = local write "dy"(w513) -> ()
                          }
                        }
                      }
                    }
                  }
                }
                n332 = Unregister For Events(event registration refnum=w394) -> ()  [unwired: 1 in, 1 out]
              }
              frame #3 {
                n333 = property on="Abort Multi Grab" class="Bool"("DisabledEnum"=T2."Disabled and Grayed Out" ("Disabled")) -> ()  [unwired: 2 in, 2 out]
                n334 = property on="Multi Grab" class="Bool"("DisabledEnum"=T2."Enabled" ("Disabled")) -> ()  [unwired: 2 in, 2 out]
              }
            }
          }
          event "Stop": Value Change {
            n335 = event-data() -> ()  [unwired: 1 in, 6 out]
            n336 = flat-sequence {
              tunnel: w533 -> [w535]
              tunnel: w530 -> [w534]
              tunnel: [w537] -> w532
              tunnel: w530 -> [w536]
              frame #0 {
                n337 = call "QI_CloseCam.vi"("Camera Handle"=w535, "path to dll"=w534) -> ()  [unwired: 1 in, 3 out]
              }
              frame #1 {
                n338 = call "QI_CloseLib.vi"("path to dll"=w536) -> ("error out"=w537:errorcluster)  [unwired: 1 in, 1 out]
              }
            }
          }
          event "Exposure Time (µs)": Value Change {
            n339 = event-data() -> ()  [unwired: 1 in, 6 out]
            n340 = property on="Exposure Time (µs)" class="DigNum (strict)"() -> ("Value"=w542:u32)  [unwired: 2 in, 2 out]
            n341 = call "QI_ConfigCam.vi"("Camera Handle"=w541, "Parameter"=Parameter."Exposure", "paramVal"=w542, "error in (no error)"=w540, "path to dll"=w538) -> ("error out"=w539:errorcluster)  [unwired: 12 in, 2 out]
          }
          event "Binning": Value Change {
            w550 = Parameter."Binning" ("Parameter")
            n342 = event-data() -> ("NewVal"=w549:u32)  [unwired: 1 in, 5 out]
            n343 = property on="CCD Height" class="DigNum (strict)"() -> ("Value"=w547:u32)  [unwired: 2 in, 2 out]
            n344 = property on="CCD Width" class="DigNum (strict)"() -> ("Value"=w548:u32)  [unwired: 2 in, 2 out]
            n345 = call "QI_ConfigCam.vi"("Camera Handle"=w560, "Parameter"=w550, "paramVal"=w549, "error in (no error)"=w559, "path to dll"=w544, "CCD Width"=w548, "CCD Height"=w547) -> ("Camera Handle"=w551:u32, "error out"=w552:errorcluster)  [unwired: 10 in, 1 out]
            n346 = call "QI_ConfigCam.vi"("Camera Handle"=w551, "Parameter"=w550, "paramVal"=w549, "error in (no error)"=w552, "path to dll"=w544, "CCD Width"=w548, "CCD Height"=w547) -> ("Camera Handle"=w546:u32, "error out"=w545:errorcluster)  [unwired: 10 in, 1 out]
            n347 = for {
              N: 6 -> [_]
              shift-right: [w567] -> w558
              shift-left: w545 -> [w571]
              tunnel: [w566] -> _
              tunnel: [w565] -> w557 mode=indexing
              tunnel: [w564] -> _ mode=indexing
              tunnel: w546 -> [w563]
              tunnel: w544 -> [w562]
              i -> [w570]
              n348 = Add(x=u32 8, y=w570) -> (x+y=w568:u32)
              n349 = call "QI_GetCamInfo.vi"("path to dll"=w562, "error in (no error)"=w571, "paramKey"=w568, "Camera Handle"=w563) -> ("error out"=w567:errorcluster, "CamInfo err"=w564:i32, "paramVal"=w565:u32, "Camera Handle"=w566:u32)  [unwired: 4 in]
            }
            n350 = Index Array(array=w557, index #1=0 ("index"), index #2=1 ("index")) -> (element #1=w553:u32, element #2=w554:u32)
            n351 = property on="ParamVal" class="Arr (strict)"("Value"=w557) -> ()  [unwired: 2 in, 2 out]
            n352 = property on="ROI Height" class="DigNum (strict)"("Value"=w554) -> ()  [unwired: 2 in, 2 out]
            n353 = property on="ROI Width" class="DigNum (strict)"("Value"=w553) -> ()  [unwired: 2 in, 2 out]
          }
          event "Trig": Value Change {
            n354 = event-data() -> ("NewVal"=w577:bool)  [unwired: 1 in, 5 out]
            n355 = Boolean To (0,1)(Boolean=w577) -> (0, 1=w578:i16)
            n356 = To Unsigned Long Integer(number=w578) -> (unsigned 32bit integer=w575:u32)
            n357 = call "QI_ConfigCam.vi"("Camera Handle"=w574, "Parameter"=Parameter."Trigger Type", "paramVal"=w575, "error in (no error)"=w576, "path to dll"=w572) -> ("error out"=w573:errorcluster)  [unwired: 12 in, 2 out]
          }
          event "Captured Image": Mouse Down {
            n358 = event-data() -> ("Coords.Horizontal"=w581:i32, "Coords.Vertical"=w580:i32, "Button"=w585:u16, "Mods.Double Click"=w586:bool)  [unwired: 1 in]
            n359 = control-ref of="Captured Image"() -> (w582:refnum<vi>)
            n360 = Select(t=w585, s=w586, f=u16 0) -> (s? t:f=w583:u16)
            n361 = case shown="1, 3" w583 {
              selector: w583 -> [_ w594]
              tunnel: w582 -> [_ w587]
              tunnel: w581 -> [_ w601]
              tunnel: w580 -> [_ w600]
              frame 0, Default {
              }
              frame 1, 3 {
                n362 = Equal?(x=w594, y=u16 1) -> (x = y?=w592:bool)
                n363 = call "mousePositinToCursorPoistion.vi"("Mouse Y position"=w600, "Mouse X position"=w601, "reference"=w587) -> ("Cursor Y position"=w599:dbl, "Cursor X position"=w598:dbl, "reference out"=w597:refnum<vi>)  [unwired: 1 in, 1 out]
                n364 = Select(t=u16 0, s=w592, f=u16 1) -> (s? t:f=w591:u16)
                n365 = call "changeCursorPosition.vi"("Cursor Y position"=w599, "Cursor X position"=w598, "Cursos id"=w591, "reference"=w597) -> ("error out"=w596:errorcluster, "reference out"=w595:refnum<vi>)  [unwired: 2 in]
                n366 = call "getDyOfCursors.vi"("error in (no error)"=w596, "reference"=w595) -> ("dy"=w588:dbl)  [unwired: 7 in, 2 out]
                n367 = local write "dy"(w588) -> ()
              }
            }
          }
        }
        n368 = Compound Arithmetic op=OR(w122, w121) -> (w123:bool)
      }
    }
  }
  n369 = property on="Camera Handle" class="DigNum (strict)"() -> ("Value"=w2:u32)  [unwired: 2 in, 2 out]
  n370 = call "QI_ToggleStreaming.vi"("Enable?"=enum16{"Disable", "Enable"}."Disable", "Camera Handle"=w2) -> ("enable"=w4:u32)  [unwired: 6 in, 3 out]
  n371 = Not Equal To 0?(x=w4) -> (x != 0?=w3:bool)
  n372 = property on="Waiting for Trigger" class="Bool (strict)"("Value"=w3) -> ()  [unwired: 2 in, 2 out]
  n373 = flat-sequence {
    tunnel: w5 -> [w603]
    frame #0 {
      n374 = property on="Stop" class="Bool (strict)"("Value"=FALSE ("Stop")) -> ()  [unwired: 2 in, 2 out]
      n375 = property on="error out" class="Clust (strict)"("Value"=w603) -> ()  [unwired: 2 in, 2 out]
    }
  }
